vi "GINKGO - MTMP - 20180213A.vi"() -> ()   [LabVIEW 2015]
uses:
  <vilib>/rvi/interface/nirviMethod/nirviMethod.xnode
  <vilib>/rvi/interface/nirviCloseFPGA/nirviCloseFPGA.xnode
  <vilib>/rvi/interface/nirviReadWriteControl/nirviReadWriteControl.xnode
  <vilib>/rvi/interface/nirviOpenFPGA/nirviOpenFPGA.xnode
  <vilib>/rvi/interface/Simulation/niFpgaSimulationCallBeginRW.vi
  <vilib>/rvi/errors/niLvFpgaAdjustHostInterfaceError.vi
  <vilib>/rvi/errors/niLvFpgaMergeErrorWithErrorCode.vi
  <vilib>/FPGAPlugInAG/Dynamic/niLvFpga_Abort_Dynamic.vi
  <vilib>/FPGAPlugInAG/Dynamic/niLvFpga_Reset_Dynamic.vi
  <vilib>/FPGAPlugInAG/Dynamic/niLvFpga_Run_Dynamic.vi
  NiFpgaLv.dll
  <vilib>/Utility/error.llb/Error Cluster From Error Code.vi
  <vilib>/FPGAPlugInAG/Dynamic/niLvFpga_Close_Dynamic.vi
  <vilib>/FPGAPlugInAG/Dynamic/niLvFpga_ReadFifo_Dynamic.vi
  <vilib>/rvi/interface/common/dynamic/niFpgaDynamicAddResources.vi
  <vilib>/FPGAPlugInAG/Dynamic/niLvFpga_StopFifo_Dynamic.vi
  Controls/Save picture camera.vi
  <vilib>/vision/NI_Vision_Development_Module.lvlib
  Global Variable/GV_Z axis.vi
  Global Variable/GV_Lock State.vi
  <vilib>/FPGAPlugInAG/Dynamic/niLvFpga_WriteFifo_Dynamic.vi
  <vilib>/FPGAPlugInAG/Dynamic/niLvFpga_ConfigureFifo_Dynamic.vi
  <vilib>/FPGAPlugInAG/Dynamic/niLvFpga_StartFifo_Dynamic.vi
  FPGA Bitfiles/MiniScan2.2.9_7853R_FPGAControl5_Gcp--B4KBuM.lvbitx
  FPGA/FPGA Control.vi
  FPGA Bitfiles/MiniScan2.2.9_7961R_FPGA796xR2_XT1A-d32QCQ.lvbitx
  FPGA/FPGA 796xR.vi
  FPGA Bitfiles/GINKGO-MTPM_7854R_FPGAControl5_d88-Mrxru6Q.lvbitx
  <vilib>/FPGAPlugInAG/PXI-7854R/niLvFpga_Open_PXI-7854R.vi
  FPGA Bitfiles/GINKGO-MTPM_7975R_FPGA796xR_a2zTekeNlbw.lvbitx
  <vilib>/FPGAPlugInAG/PXIe-7975R/niLvFpga_Open_PXIe-7975R.vi
  <vilib>/FPGAPlugInAG/PXI-7853R/niLvFpga_Open_PXI-7853R.vi
  <vilib>/FPGAPlugInAG/PXIe-7961R/niLvFpga_Open_PXIe-7961R.vi
panel:
  out "波形图表":sgl(graph)=113.25391
  in  "ROI Statistic":bool=TRUE
  out "Mean Value":sgl=113.25391
  out "Variation":sgl=54.35391
  out "Minimal":sgl=32720.0
  out "Maximal":sgl=33176.0
  out "Power Stop":bool=TRUE
  in  "Rolling Queue Flag":bool=TRUE
  out "Total Data Out":u16=13612
  in  "Acq. Start":u16=38 caption="Phase" max=6000 step=1
  in  "Real Back Period":u16=5 min=1
  out "实际深度":u32=8388608
  in  "Map Max.":i32=10000 caption="Max."
  in  "Map Min.":i32=-500 caption="Min."
  out "Scale Value":dbl=0.1 caption="X"
  out "Total Frames":u16=16553
  in  "Max. Min.":cluster{i32, i32}(slide)={429, -176} scale=-500.0..10000.0
  in  "16-bit Display Method":u32(ring)=14 caption="Display Method" items=["Full Dynamic"=12, "Given Range"=14]
  in  "Rolling Average":dbl=2.0 min=1.0 step=1.0
  in  "Rolling":bool=TRUE
  out "User Define Phase":u32=746
  out "Image":T1(plugin-control)
  in  "Controls":T2(tab)
  in  "Start Device":bool
  in  "PMT Shutter Pow.":bool
  out "Overload Dis.":bool=TRUE
  in  "Pulse Number":enum16{"SP", "DP"}(ring)
  in  "Mems Enable":bool
  out "中心偏移":i32
  in  "互相关点数":i32=5
  in  "Calculate Phase shift":bool
  in  "Wave":enum16{"Triangle", "Sine", "Ramp"}(ring)=enum."Sine"
  in  "Interval Dis.":sgl=0.00049965957 min=-10 max=50 format="%.4f"
  in  "stop z stage":bool
  in  "5V":bool
  in  "Voltage Level":dbl=15.0 format="%#.3p"
  in  "Voltage Level 2":dbl=-15.0 caption="Voltage Level" format="%#.3p"
  in  "Source:Output Enabled":bool
  out "Voltage Measurement 2":dbl=-0.0001217159676001422 caption="Voltage Measurement"
  out "Compliance/Limit Reached 2":bool caption="Compliance/Limit Reached"
  out "Voltage Measurement":i8
  out "Compliance/Limit Reached":bool
  in  "MEMS SLOW":dbl(slide)=240000.0 caption="Slow" min=0.0 max=1000000.0 step=100.0 scale=0.0..300000.0 scale format="%#_6p"
  in  "MEMS FAST":dbl(slide) caption="Fast" min=0.0 max=1000000.0 step=100.0 scale=0.0..300000.0 scale format="%#_6p"
  out "Stimulate Time Dis.":u32
  in  "Stimulate Value":dbl=5.0 min=-10.0 max=10.0 format="%#_3f"
  in  "Stimulate Time":u32=500
  out "Stimulate Interval Time":dbl=1.9692307692307693
  in  "Stimulate Interval":u32=10
  in  "Stimulate Enable":bool caption="V.S."
  out "Frame Befor Time":dbl=845778175.0153847
  out "Frame Number":u32=4294967295
  in  "Frames Befor Stimulate":u32
  out "Acq. Sample Rate":dbl=120000000.0 caption="Sanple Rate Divider" format="%#_6p"
  in  "Microscope":enum16{"Miniature", "Benchtop"}(ring)
  in  "Line":u32(ring)=512 caption="Y" items=["8"=8, "16"=16, "32"=32, "64"=64, "128"=128, "256"=256, "512"=512, "1024"=1024, "2048"=2048]
  in  "X Offset":dbl caption="X" format="%#_3f"
  in  "Y Offset":dbl caption="Y" min=-10.0 max=10.0 format="%#_3f"
  in  "X Frequency":dbl(slide)=2600.0 caption="Speed" min=50.0 max=10000.0 step=1.0 scale=0.0..5000.0
  in  "Laser Intensity":dbl(slide)=2.0786516853932584 max=10.0 scale=0.0..5.0
  in  "Phase Shift":u32(slide)=752 caption="Phase" max=15000 step=2 scale=0.0..15000.0
  in  "Point":bool
  in  "PMT1 Sensitivity":dbl(slide)=0.5 min=0.0 max=0.95 step=0.05 scale=0.0..0.95 scale format="%#_3f"
  in  "PMT1 Enable":bool=TRUE
  out "Pixel Dwell":dbl=0.2988 format="%#_3g"
  out "Actual Positon":sgl=11.119017
  out "Actual Laser Intensity":dbl(knob)=0.69488525390625 scale=-10.0..1.0
  in  "PMT2 Switch":bool
  in  "PMT2 Sensitivity":dbl(slide)=0.45 min=0.0 max=0.95 step=0.05 scale=0.0..0.95 scale format="%#_3f"
  in  "File Name":string
  in  "Scale":bool
  in  "XY Home":bool
  in  "XY UP":bool
  in  "XY DOWN":bool
  in  "XY LEFT":bool
  in  "XY RIGHT":bool
  in  "Stop":bool=TRUE
  in  "LIVE":bool
  in  "Save":bool
  in  "Z-Stack":bool
  in  "Pixel/Line":u16(ring)=512 caption="X" items=["8"=8, "16"=16, "32"=32, "64"=64, "128"=128, "256"=256, "512"=512, "1024"=1024, "2048"=2048]
  in  "Gain":enum16{"0dB", "6dB", "12dB"}(ring)
  in  "Coulple":enum16{"AC", "DC"}(ring)=enum."DC"
  in  "Path":path=path "C:/Users/TVS001/Desktop/DATA/20180207/13-zz-gcamp" caption="Images Folder"
  out "Save Frames Dis.":u16=1000
  in  "Save Frames":u16=1000
  in  "ZOOM":u16(ring)=2 items=["User Define", "1X", "1.5X", "2X", "2.5X", "3X", "3.5X", "4X", "4.5X", "5X", "6X"]
  in  "Scan Mode":enum16{"Normal", "Line Scan", "Random Access"}(ring)
  in  "Y Amplitude":dbl=0.6 caption="Y" min=-10.0 max=18.0 format="%0.2p"
  in  "X Amplitude":dbl=0.6 caption="X" min=-10.0 max=18.0 format="%.2p"
  in  "Add Phase":bool
  in  "Move":bool=TRUE
  out "Frame Rate":dbl=5.078125 format="%#_3g"
  out "Ready":u8(slide)=10 scale=0.0..10.0
  in  "Z":bool
  out "Position":sgl=-5.9652176 format="%#_6f"
  in  "Set Zero":bool caption="空白按钮"
  in  "Reset Zero":bool caption="空白按钮"
  in  "Home Z":bool
  in  "Abs. Go":bool
  in  "Abs Pos X":sgl min=-10 max=360 format="%.6f"
  in  "Z Up":bool
  in  "Z Down":bool
  in  "Jog":sgl=0.0005 caption="Z" min=0 max=50 step=0.0001 format="%.4f"
  in  "Frames/Slice":u16=5
  in  "Slices":u16=87
  out "End Dis.":sgl=0.043470383 format="%#_6f"
  out "Start Dis.":sgl format="%#_6f"
  in  "End":bool
  in  "Start":bool
  in  "Restart":bool
  in  "Interval Time":u32=150
  in  "Zoom Standard":dbl[][](array[numeric])=[[10.0, 10.0, 11251.0], [6.66, 6.66, 10603.0], [5.0, 5.0, 10394.0], [4.0, 4.0, 10394.0], [3.34, 3.34, 8602.0], [2.86, 2.86, 10394.0], [2.5, 2.5, 10394.0], [2.222, 2.222, 10394.0], [1.3, 1.3, 8294.0], [0.6, 0.6, 8296.0]]
  in  "Zoom Miniature":dbl[][](array[numeric])=[[14.0, 8.0, 738.0], [12.0, 7.0, 746.0], [9.0, 6.0, 752.0], [7.2, 5.6, 754.0], [5.0, 4.0, 738.0], [5.14, 4.0, 846.0], [4.0, 3.0, 744.0], [3.6, 2.0, 840.0], [3.2, 2.3, 754.0], [3.0, 2.33, 740.0]]
  out "Test Point2":u32
  out "Test Point 3":u32=143394
  out "Test Point":u32
  out "Point/Pixel":i32=36
  in  "Focus Flag":bool
  out "Queue Number":i32=2
  out "Initial Z":bool
  out "Initialization Done":bool=TRUE
  in  "Start Control":bool
  out "Memory":i32(slide) scale=0.0..5000.0
  in  "Resource Name":refnum<k15>="PXI1Slot6"
  in  "Channel Name":string="1" caption="Channel Name 1"
  in  "Current Limit":dbl=0.5 format="%.3p"
  in  "Voltage Level Range":dbl=20.0 format="%.5p"
  in  "Current Limit Range":dbl=1.0 format="%.3p"
  in  "Source Delay (Sec)":dbl=0.1 format="%.3p"
  in  "Channel Name 2":string="2"
  out "Current Measurement 2":dbl=-3.1048749529460624e-06 caption="Current Measurement"
  out "Current Measurement":i16
  out "Actual DDS Ticks":u32=1
  out "Actual DDS Sample Freq":u32=279173
  in  "OUTPUT Value Ticks":u32=44
  in  "DDS Ticks":u32=1
  out "Actual OUTPUT Value Ticks":u32=44
  in  "Random 1D Array":fxp<+/-,32,16>[](array[numeric]) format="%.21g"
  in  "MG17Motor Z":refnum<k7>(container)
  out "Acq. Point Dis.":u16=32
  in  "Divide":enum16{"120M", "60M", "30M", "15M", "7.5M"}(ring)
  out "Nonlinear Acq.":bool=TRUE
  in  "Adapter Module User Data 1":u8
  in  "Adapter Module User Data 0":u8
  in  "Adapter Module User Command":u8=3
  in  "Apply":bool
  in  "HWSerialNum":i32=49871607
  in  "Set Large Scale":dbl=0.5 caption="X"
  in  "Set Small Scale":dbl=0.1 caption="X"
  in  "Set Zero Value":sgl format="%#_6f"
  in  "Fill Fraction":dbl=0.8 min=0.1 max=6.0 step=0.01
  in  "Back Period":u16=5 min=1
  in  "Initial Benchtop Speed":dbl=500.0 caption="Speed" min=50.0 max=10000.0 step=1.0
  in  "Initial Miniature Speed":dbl=2600.0 caption="Speed" min=50.0 max=10000.0 step=1.0
  out "Acq.Point Array":u16[](graph)=[38, 38, 38, 37, 37, 37, 37, 36, 36, 36, 36, 36, 35, 35, 35, 35, 35, 34, 34, 34, 34, 34, 34, 33, 33, 33, 33, 33, 33, 32, 32, 32, 32, 32, 32, 32, 32, 31, 31, 31, 31, 31, 31, 31, 31, 30, 30, 30, 30, 30, 30, 30, 30, 30, 30, 29, 29, 29, 29, 29, 29, 29, 29, 29, 29, 29, 28, 28, 28, 28, 28, 28, 28, 28, 28, 28, 28, 28, 28, 28, 27, 27, 27, 27, 27, 27, 27, 27, 27, 27, 27, 27, 27, 27, 27, 27, 26, 26, 26, 26, 26, 26, 26, 26, 26, 26, 26, 26, 26, 26, 26, 26, 26, 26, 26, 26, 26, 25, 25, 25, 25, 25, 25, 25, 25, 25, 25, 25, 25, 25, 25, 25, 25, 25, 25, 25, 25, 25, 25, 25, 25, 25, 25, 25, 24, 24, 24, 24, 24, 24, 24, 24, 24, 24, 24, 24, 24, 24, 24, 24, 24, 24, 24, 24, 24, 24, 24, 24, 24, 24, 24, 24, 24, 24, 24, 24, 24, 24, 24, 24, 24, 24, 24, 24, 24, 24, 24, 23, 23, 23, 23, 23, 23, 23, 23, 23, 23, 23, 23, 23, 23, 23, 23, 23, 23, 23, 23, 23, 23, 23, 23, 23, 23, 23, 23, 23, 23, 23, 23, 23, 23, 23, 23, 23, 23, 23, 23, 23, 23, 23, 23, 23, 23, 23, 23, 23, 23, 23, 23, 23, 23, 23, 23, 23, 23, 23, 23, 23, 23, 23, 23, 23, 23, 23, 23, 23, 23, 23, 23, 23, 23, 23, 23, 23, 23, 23, 23, 23, 23, 23, 23, 23, 23, 23, 23, 23, 23, 23, 23, 23, 23, 23, 23, 23, 23, 23, 23, 23, 23, 23, 23, 23, 23, 23, 23, 23, 23, 23, 23, 23, 23, 23, 23, 23, 23, 23, 23, 23, 23, 23, 23, 23, 23, 23, 23, 23, 23, 23, 23, 23, 23, 23, 23, 23, 23, 24, 24, 24, 24, 24, 24, 24, 24, 24, 24, 24, 24, 24, 24, 24, 24, 24, 24, 24, 24, 24, 24, 24, 24, 24, 24, 24, 24, 24, 24, 24, 24, 24, 24, 24, 24, 24, 24, 24, 24, 24, 24, 24, 25, 25, 25, 25, 25, 25, 25, 25, 25, 25, 25, 25, 25, 25, 25, 25, 25, 25, 25, 25, 25, 25, 25, 25, 25, 25, 25, 26, 26, 26, 26, 26, 26, 26, 26, 26, 26, 26, 26, 26, 26, 26, 26, 26, 26, 26, 26, 26, 27, 27, 27, 27, 27, 27, 27, 27, 27, 27, 27, 27, 27, 27, 27, 27, 28, 28, 28, 28, 28, 28, 28, 28, 28, 28, 28, 28, 28, 28, 29, 29, 29, 29, 29, 29, 29, 29, 29, 29, 29, 30, 30, 30, 30, 30, 30, 30, 30, 30, 30, 31, 31, 31, 31, 31, 31, 31, 31, 32, 32, 32, 32, 32, 32, 32, 32, 33, 33, 33, 33, 33, 33, 34, 34, 34, 34, 34, 34, 35, 35, 35, 35, 35, 36, 36, 36, 36, 36, 37, 37, 37, 37, 38, 38, 38]
  out "Init Data Out":u16[](array[numeric])=[38, 38, 38, 37, 37, 37, 37, 36, 36, 36, 36, 36, 35, 35, 35, 35, 35, 34, 34, 34, 34, 34, 34, 33, 33, 33, 33, 33, 33, 32, 32, 32, 32, 32, 32, 32, 32, 31, 31, 31, 31, 31, 31, 31, 31, 30, 30, 30, 30, 30, 30, 30, 30, 30, 30, 29, 29, 29, 29, 29, 29, 29, 29, 29, 29, 29, 28, 28, 28, 28, 28, 28, 28, 28, 28, 28, 28, 28, 28, 28, 27, 27, 27, 27, 27, 27, 27, 27, 27, 27, 27, 27, 27, 27, 27, 27, 26, 26, 26, 26, 26, 26, 26, 26, 26, 26, 26, 26, 26, 26, 26, 26, 26, 26, 26, 26, 26, 25, 25, 25, 25, 25, 25, 25, 25, 25, 25, 25, 25, 25, 25, 25, 25, 25, 25, 25, 25, 25, 25, 25, 25, 25, 25, 25, 24, 24, 24, 24, 24, 24, 24, 24, 24, 24, 24, 24, 24, 24, 24, 24, 24, 24, 24, 24, 24, 24, 24, 24, 24, 24, 24, 24, 24, 24, 24, 24, 24, 24, 24, 24, 24, 24, 24, 24, 24, 24, 24, 23, 23, 23, 23, 23, 23, 23, 23, 23, 23, 23, 23, 23, 23, 23, 23, 23, 23, 23, 23, 23, 23, 23, 23, 23, 23, 23, 23, 23, 23, 23, 23, 23, 23, 23, 23, 23, 23, 23, 23, 23, 23, 23, 23, 23, 23, 23, 23, 23, 23, 23, 23, 23, 23, 23, 23, 23, 23, 23, 23, 23, 23, 23, 23, 23, 23, 23, 23, 23, 23, 23, 23, 23, 23, 23, 23, 23, 23, 23, 23, 23, 23, 23, 23, 23, 23, 23, 23, 23, 23, 23, 23, 23, 23, 23, 23, 23, 23, 23, 23, 23, 23, 23, 23, 23, 23, 23, 23, 23, 23, 23, 23, 23, 23, 23, 23, 23, 23, 23, 23, 23, 23, 23, 23, 23, 23, 23, 23, 23, 23, 23, 23, 23, 23, 23, 23, 23, 23, 24, 24, 24, 24, 24, 24, 24, 24, 24, 24, 24, 24, 24, 24, 24, 24, 24, 24, 24, 24, 24, 24, 24, 24, 24, 24, 24, 24, 24, 24, 24, 24, 24, 24, 24, 24, 24, 24, 24, 24, 24, 24, 24, 25, 25, 25, 25, 25, 25, 25, 25, 25, 25, 25, 25, 25, 25, 25, 25, 25, 25, 25, 25, 25, 25, 25, 25, 25, 25, 25, 26, 26, 26, 26, 26, 26, 26, 26, 26, 26, 26, 26, 26, 26, 26, 26, 26, 26, 26, 26, 26, 27, 27, 27, 27, 27, 27, 27, 27, 27, 27, 27, 27, 27, 27, 27, 27, 28, 28, 28, 28, 28, 28, 28, 28, 28, 28, 28, 28, 28, 28, 29, 29, 29, 29, 29, 29, 29, 29, 29, 29, 29, 30, 30, 30, 30, 30, 30, 30, 30, 30, 30, 31, 31, 31, 31, 31, 31, 31, 31, 32, 32, 32, 32, 32, 32, 32, 32, 33, 33, 33, 33, 33, 33, 34, 34, 34, 34, 34, 34, 35, 35, 35, 35, 35, 36, 36, 36, 36, 36, 37, 37, 37, 37, 38, 38, 38]
  out "x amp. new":dbl
  out "y amp. new":dbl
  in  "Add Random Access":bool
  out "x offset new":i16=-7638
  out "y offset new":i16=-4030
  in  "All Random Array":fxp<+/-,32,16>[][](array[numeric])
  in  "Clear Array":bool
  out "Random Phase":u32=12 caption="Phase" max=6000 step=1
  # "File Name"
  # "File Path"
  # "Save Frames"
  # "Microscope"
  # "Scan Mode"
  # "PMT1"
  # "PMT2"
  # "Frame Size"
  # "Gain"
  # "Scan Speed"
  # "Hz"
  # "V"
  # "V"
  # "Rate"
  # "Frame Rate"
  # "μs"
  # "Hz"
  # "Pixel Dwell"
  # "XY"
  # "Z"
  # "Zoom"
  # "Point"
  # "Amplitude"
  # "V"
  # "V"
  # "Phase"
  # "Laser"
  # "Intensity Map"
  # "Recent Z"
  # "Frames Before"
  # "s"
  # "Stimulate Interval"
  # "s"
  # "ms"
  # "Stimulate Time"
  # "V"
  # "Stimulate Intensity"
  # "Mode Switch"
  # "MEMS Filter"
  # "Acquisition Mode"
  # "Image Settings"
  # "Magnification"
  # "Save Settings"
  # "Position Settings"
  # "Detection Settings"
  # "Z-scan Settings"
  # "Vision Stimulate Settings"
  # "X"
  # "Y"
  # "Phase"
  # "1X"
  # "1.5X"
  # "2X"
  # "2.5X"
  # "3X"
  # "3.5X"
  # "4X"
  # "4.5X"
  # "5X"
  # "6X"
  # "X"
  # "Y"
  # "Phase"
  # "1X"
  # "1.5X"
  # "2X"
  # "2.5X"
  # "3X"
  # "3.5X"
  # "4X"
  # "4.5X"
  # "5X"
  # "6X"
  # "40859011"
  # "83856379"
  # "AO0 -- X-Miniature  \nAO1 -- Y-Miniature\nAO2 -- Laser Intensity\nAO3 -- PMT1\nAO4 -- PMT2 \nAO5 -- \nAO6 -- X-Benchtop\nAO7 -- Y-Benchtop\n\nAI0  -- Actual Laser Intensity"
  # "DIO0 -- Acqusition  \nDIO1 -- VSYNC\nDIO2 -- HSYNC \nDIO3 -- Laser Shutter\nDIO4 -- MEMS FAST Filter\nDIO5 -- MEMS SLOW Filter\nDIO6 -- PMT Shutter\nDIO7 -- PMT Shutter Pow.\nDIO8 -- Shock Detection \nDIO9 -- Foot-plate LIVE Detection"
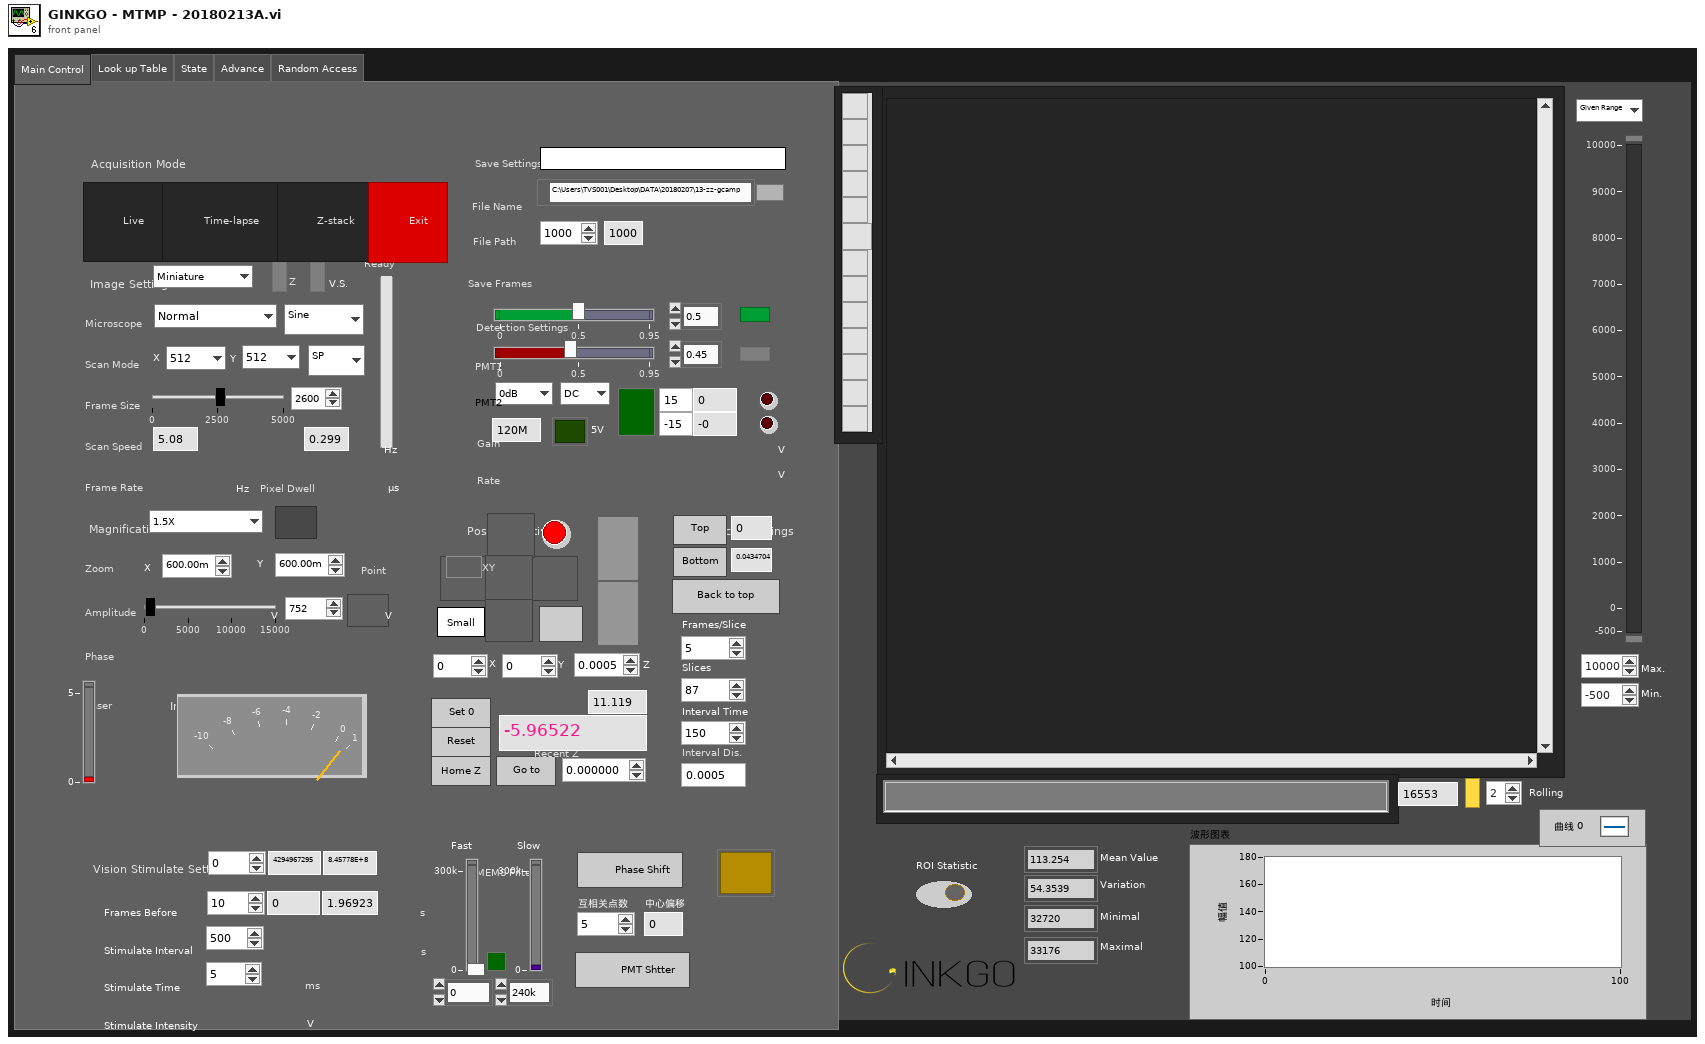
[diagram p1: front panel]
types:
  T1 = typedef "IMAQ Image.ctl" = refnum<image>
  T2 = enum32{"Main Control", "Look up Table", "State", "Advance", "Random Access"}
  T3 = typedef "Image Type" = u32
  T4 = enum8{"Enabled", "Disabled", "Disabled and Grayed Out"}
  T5 = cluster{"Global Rectangle":i32[], "Contours":cluster{"Contour Type":u32, "ROI Type":u32, "Points":i32[]}[]}
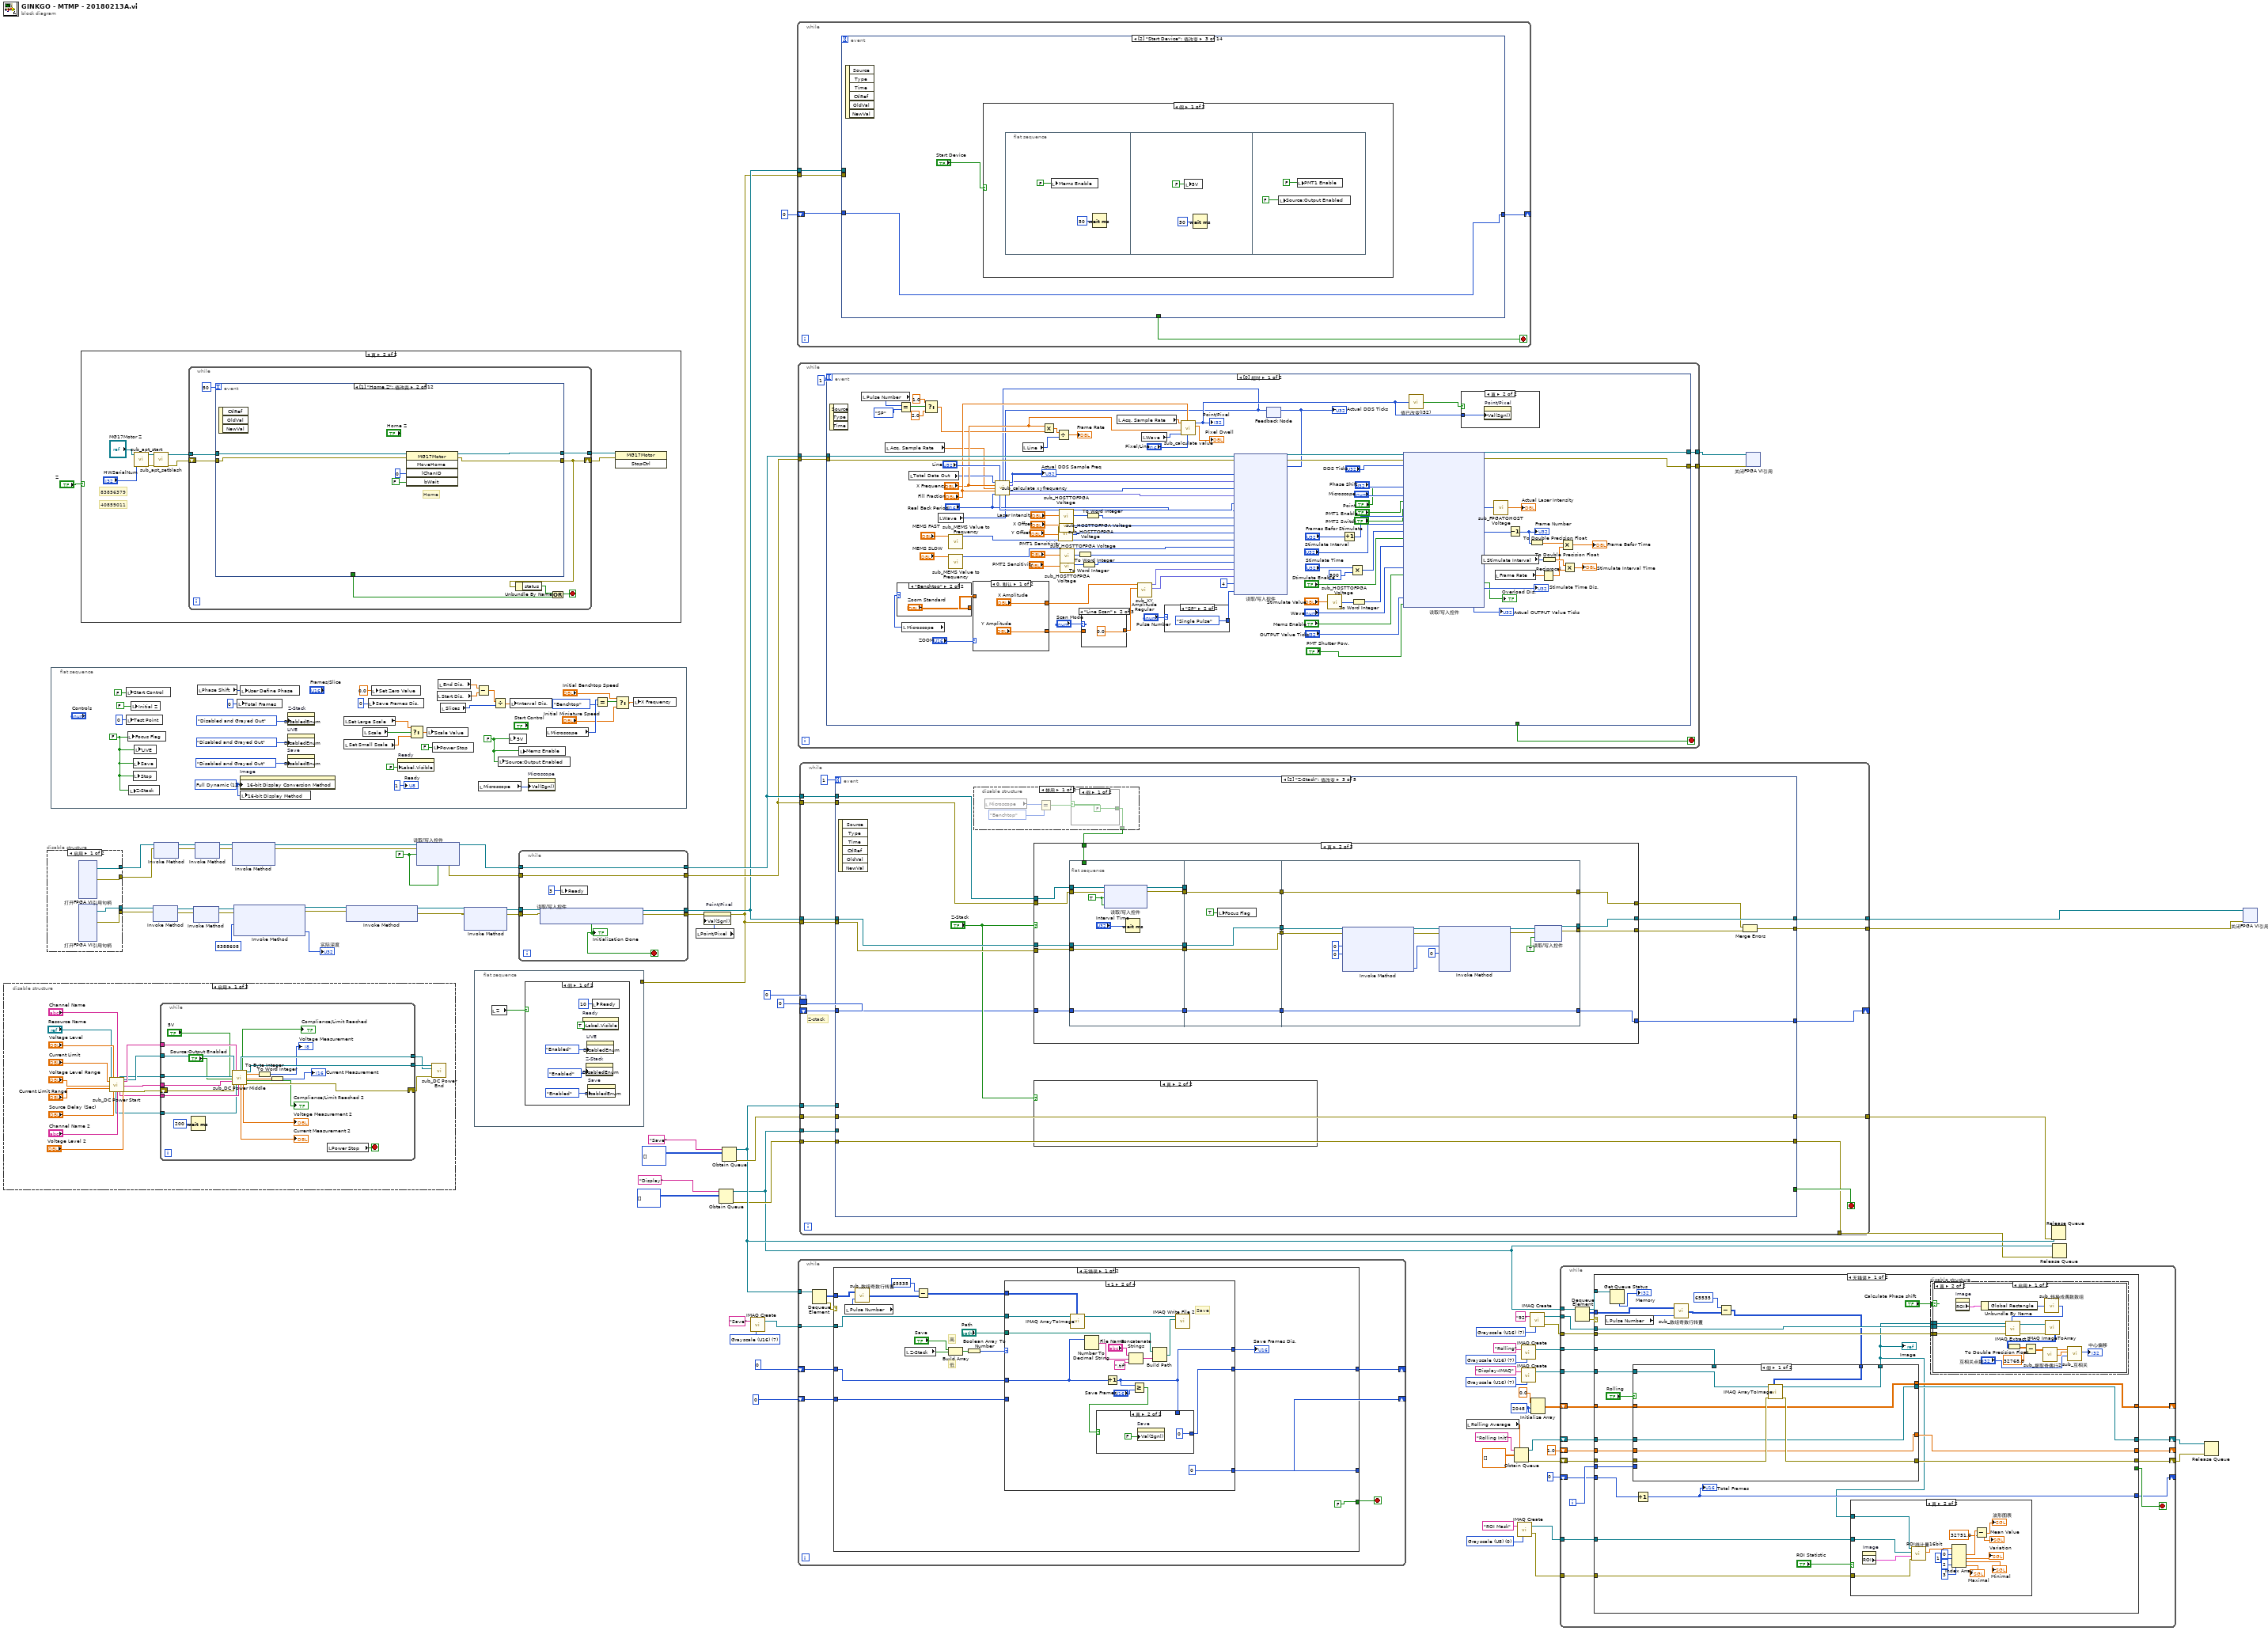
[diagram p0: block diagram]
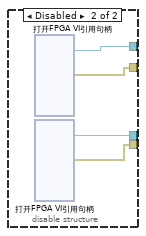
[diagram p2: hidden frame]
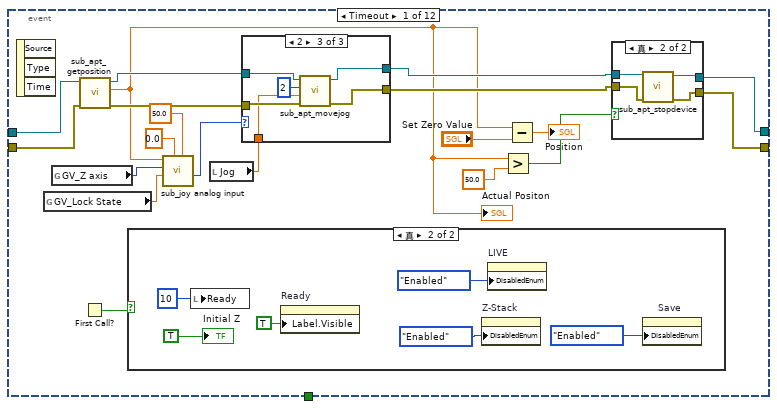
[diagram p4: hidden frame]
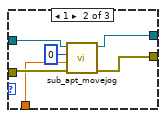
[diagram p6: hidden frame]
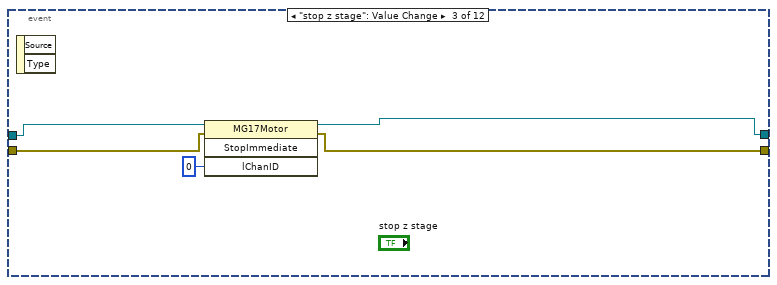
[diagram p9: hidden frame]
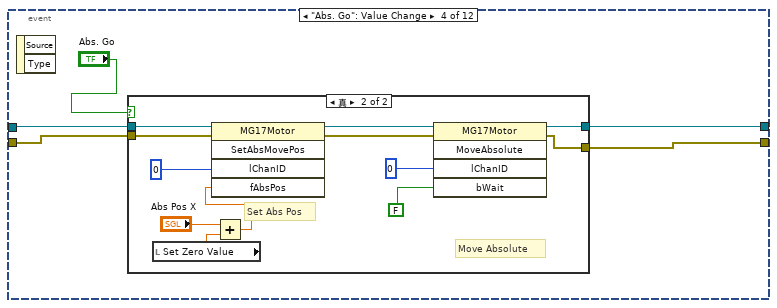
[diagram p10: hidden frame]
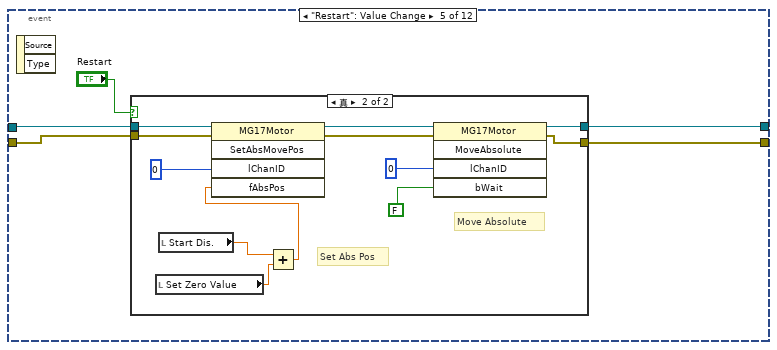
[diagram p12: hidden frame]
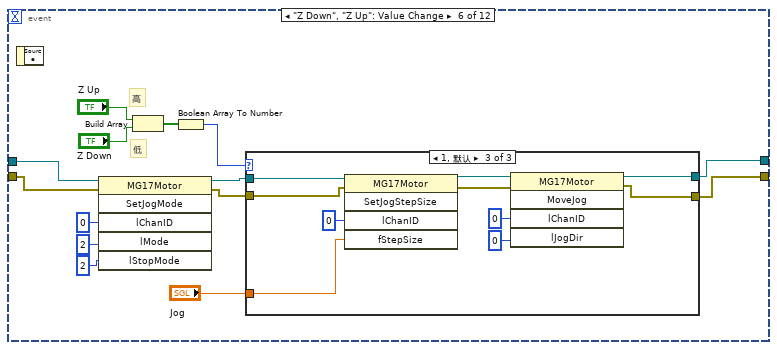
[diagram p14: hidden frame]
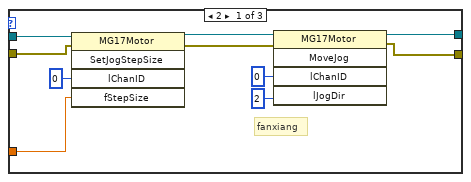
[diagram p15: hidden frame]
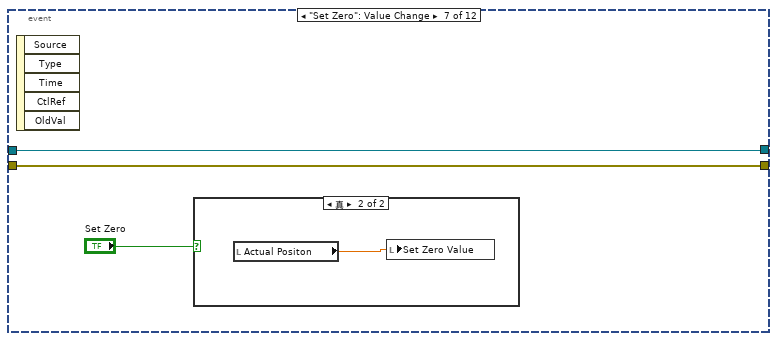
[diagram p17: hidden frame]
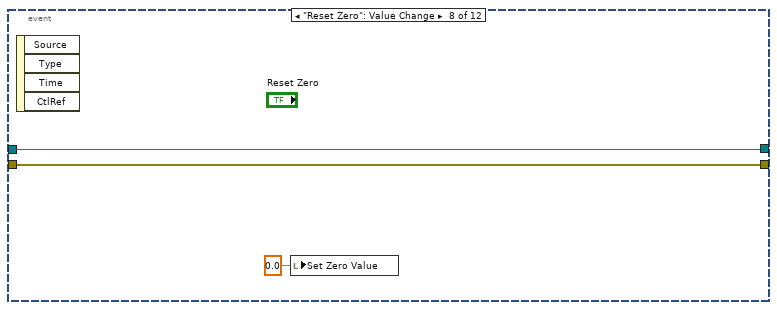
[diagram p19: hidden frame]
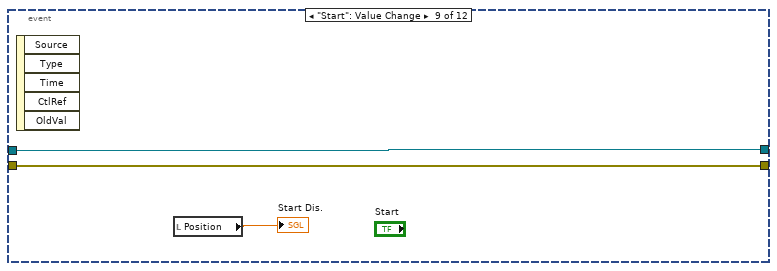
[diagram p20: hidden frame]
diagram:
  w3 = T3 0 items=["Grayscale (U8)", "Grayscale (I16)", "Grayscale (SGL)", "Complex (CSG)", "RGB (U32)", "HSL (U32)", "RGB (U64)", "Grayscale (U16)"] ("Image Type")
  w9 = T3 7 items=["Grayscale (U8)", "Grayscale (I16)", "Grayscale (SGL)", "Complex (CSG)", "RGB (U32)", "HSL (U32)", "RGB (U64)", "Grayscale (U16)"] ("Image Type")
  w15 = T3 7 items=["Grayscale (U8)", "Grayscale (I16)", "Grayscale (SGL)", "Complex (CSG)", "RGB (U32)", "HSL (U32)", "RGB (U64)", "Grayscale (U16)"] ("Image Type")
  w28 = T3 7 items=["Grayscale (U8)", "Grayscale (I16)", "Grayscale (SGL)", "Complex (CSG)", "RGB (U32)", "HSL (U32)", "RGB (U64)", "Grayscale (U16)"] ("Image Type")
  w38 = 2048 ("维数大小")
  w35 = T3 7 items=["Grayscale (U8)", "Grayscale (I16)", "Grayscale (SGL)", "Complex (CSG)", "RGB (U32)", "HSL (U32)", "RGB (U64)", "Grayscale (U16)"] ("Image Type")
  w49 = FALSE ("Enable")
  n1 = disable-structure shown="启用" {
    frame Enabled {
      n2 = call "sub_DC Power Start.vi"("IVI引用句柄输入"="Resource Name", "Current Limit"="Current Limit", "Voltage Level Range"="Voltage Level Range", "Current Limit Range"="Current Limit Range", "Voltage Level"="Voltage Level", "Source Delay (Sec)"="Source Delay (Sec)", "Channel Name"="Channel Name", "Channel Name 2"="Channel Name 2", "Voltage Level 2"="Voltage Level 2") -> ("instrument handle out 2"=w81:refnum<k15>, "instrument handle out"=w88:refnum<k15>, "Channel Name 6"=w82:string, "IVI引用句柄输出"=w96:refnum<k15>, "Channel Name 4"=w97:string, "Channel Name 3"=w90:string, "错误输出"=w87:errorcluster)  [unwired: 4 in]
      n3 = while {
        tunnel: w97 -> [w121]
        tunnel: w90 -> [w120]
        tunnel: [w119] -> w89
        shift-right: [w118] -> w86
        shift-left: w87 -> [w115]
        tunnel: w88 -> [w114]
        tunnel: w96 -> [w116]
        tunnel: [w117] -> w98
        tunnel: w82 -> [w104]
        tunnel: w81 -> [w103]
        stop <- w105 stop-if-true
        n4 = Wait (ms)(milliseconds to wait=u32 200 ("等待时间（毫秒）")) -> ()  [unwired: 1 out]
        n5 = call "sub_DC Power Middle.vi"("IVI引用句柄输入"=w116, "instrument handle out"=w114, "5V"="5V", "Source:Output Enabled"="Source:Output Enabled", "Channel Name 3"=w120, "错误输入（无错误）"=w115, "Channel Name 4"=w121, "instrument handle out 2"=w103, "Channel Name 5"=w104) -> ("instrument handle out 3"=w119:refnum<k15>, "Current Measurement 2"=→"Current Measurement 2":dbl, "Compliance/Limit Reached"=→"Compliance/Limit Reached":bool, "Voltage Measurement 2"=→"Voltage Measurement 2":dbl, "IVI引用句柄输出"=w117:refnum<k15>, "Voltage Measurement"=w111:dbl, "Current Measurement"=w110:dbl, "Compliance/Limit Reached 2"=→"Compliance/Limit Reached 2":bool, "错误输出"=w118:errorcluster)  [unwired: 2 in]
        n6 = To Byte Integer(number=w111) -> (8bit integer=→"Voltage Measurement":i8)
        n7 = To Word Integer(number=w110) -> (16bit integer=→"Current Measurement":i16)
        n8 = local read "Power Stop"() -> (w105:bool)
      }
      n9 = call "sub_DC Power End.vi"("错误输入（无错误）"=w86, "instrument handle out"=w89, "IVI引用句柄输入"=w98) -> ()  [unwired: 9 in]
    }
    frame Disabled {
    }
  }
  n10 = disable-structure shown="启用" {
    disable-tunnel: [w125 w129] -> w80
    disable-tunnel: [w124 w128] -> w79
    disable-tunnel: [w123 w126] -> w78
    disable-tunnel: [w122 w127] -> w77
    frame Enabled {
      n11 = xnode "打开FPGA VI引用句柄"() -> ("FPGA VI引用输出"=w125:refnum<k20>, "错误输出"=w124:errorcluster)  [unwired: 2 in]
      n12 = xnode "打开FPGA VI引用句柄"() -> ("FPGA VI引用输出"=w122:refnum<k20>, "错误输出"=w123:errorcluster)  [unwired: 2 in]
    }
    frame Disabled {
      n13 = xnode "打开FPGA VI引用句柄"() -> ("FPGA VI引用输出"=w129:refnum<k20>, "错误输出"=w128:errorcluster)  [unwired: 2 in]
      n14 = xnode "打开FPGA VI引用句柄"() -> ("FPGA VI引用输出"=w127:refnum<k20>, "错误输出"=w126:errorcluster)  [unwired: 2 in]
    }
  }
  n15 = flat-sequence {
    frame #0 {
      w143 = FALSE ("Focus")
      w151 = u32 12 items=["Default"=10, "Most Significant Bits"=11, "Full Dynamic"=12, "Downshift"=13, "Given Range"=14, "90% Dynamic"=15, "Given Percent Range"=16] ("16-bit Display Mapping:Conversion Method")
      w158 = FALSE ("Focus")
      n16 = local write "Start Control"(FALSE ("Initial")) -> ()
      n17 = local write "Test Point"(u32 0 ("Test Point")) -> ()
      n18 = local write "Focus Flag"(w158) -> ()
      n19 = local write "Z-Stack"(w158) -> ()
      n20 = local write "Initial Z"(FALSE ("Initial")) -> ()
      n21 = local write "Save"(w158) -> ()
      n22 = local write "Stop"(w158) -> ()
      n23 = local write "LIVE"(w158) -> ()
      n24 = local read "Phase Shift"() -> (w144:u32)
      n25 = local write "Total Frames"(u16 0 ("Total Frames")) -> ()
      n26 = property on="Image" class="ImageControl"("16-bit Display Conversion Method"=w151) -> ()  [unwired: 2 in, 2 out]
      n27 = local write "User Define Phase"(w144) -> ()
      n28 = local write "16-bit Display Method"(w151) -> ()
      n29 = property on="LIVE" class="Bool (严格)"("DisabledEnum"=T4."Disabled and Grayed Out" ("禁用")) -> ()  [unwired: 2 in, 2 out]
      n30 = property on="Save" class="Bool (严格)"("DisabledEnum"=T4."Disabled and Grayed Out" ("禁用")) -> ()  [unwired: 2 in, 2 out]
      n31 = property on="Z-Stack" class="Bool (严格)"("DisabledEnum"=T4."Disabled and Grayed Out" ("禁用")) -> ()  [unwired: 2 in, 2 out]
      n32 = local read "Set Large Scale"() -> (w150:dbl)
      n33 = local read "Set Small Scale"() -> (w149:dbl)
      n34 = local read "Scale"() -> (w148:bool)
      n35 = local write "Save Frames Dis."(u16 0 ("Save Frames Dis.")) -> ()
      n36 = local write "Set Zero Value"(sgl 0.0 ("Set Zero Value")) -> ()
      n37 = property on="Ready" class="Slide (严格)"("Label.Visible"=FALSE ("标签.可见")) -> ()  [unwired: 2 in, 2 out]
      n38 = Select(t=w150, s=w148, f=w149) -> (s? t:f=w147:dbl)
      n39 = local write "Scale Value"(w147) -> ()
      n40 = local write "Power Stop"(FALSE ("Power Stop")) -> ()
      n41 = local read "Start Dis."() -> (w140:sgl)
      n42 = local read "End Dis."() -> (w139:sgl)
      n43 = local read "Slices"() -> (w138:u16)
      n44 = Subtract(x=w139, y=w140) -> (x-y=w141:sgl)
      n45 = local read "Microscope"() -> (w137:enum16{"Miniature", "Benchtop"})
      n46 = Divide(x=w141, y=w138) -> (x/y=w142:sgl)
      n47 = local write "Source:Output Enabled"(w143) -> ()
      n48 = local write "5V"(w143) -> ()
      n49 = local write "Interval Dis."(w142) -> ()
      n50 = local write "Mems Enable"(w143) -> ()
      n51 = property on="Microscope" class="Enum (严格)"("Val(Sgnl)"=w137) -> ()  [unwired: 2 in, 2 out]
      n52 = local read "Microscope"() -> (w135:enum16{"Miniature", "Benchtop"})
      n53 = Equal?(x=w135, y=enum16{"Miniature", "Benchtop"}."Benchtop") -> (x = y?=w134:bool)
      n54 = Select(t="Initial Benchtop Speed", s=w134, f="Initial Miniature Speed") -> (s? t:f=w132:dbl)
      n55 = local write "X Frequency"(w132) -> ()
      "Ready" <- u8 1 ("Process")
    }
  }
  n56 = case shown="真" "Z" {
    frame False {
    }
    frame True {
      # "40859011"
      # "83856379"
      n57 = call "sub_apt_start.vi"("HWSerialNum"="HWSerialNum", "引用"="MG17Motor Z") -> ("错误输出"=w166:errorcluster, "引用输出"=w167:refnum<k7>)  [unwired: 8 in]
      n58 = call "sub_apt_setblash.vi"("错误输入（无错误）"=w166, "引用"=w167) -> ("错误输出"=w164:errorcluster, "引用输出"=w165:refnum<k7>)  [unwired: 8 in]
      n59 = while {
        shift-right: [w173] -> w168
        shift-left: w164 -> [w176]
        tunnel: w165 -> [w177]
        tunnel: [w175] -> w169
        stop <- w171 stop-if-true
        n60 = event shown="[1] \"Home Z\": 值改变" {
          selector: _ -> [_ _ _ _ _ _ _ _ _ _ _ _]
          dyn-events: _ -> [_ _ _ _ _ _ _ _ _ _ _ _]
          timeout: 50 -> [_ _ _ _ _ _ _ _ _ _ _ _]
          tunnel: w177 -> [w190 w225 w233 w239 w258 w278 w311 w315 w318 w321 w324 w357]
          tunnel: w176 -> [w189 w224 w232 w238 w257 w277 w310 w314 w317 w320 w323 w356]
          tunnel: [w195 w227 w231 w237 w256 w286 w311 w315 w318 w321 w333 w357] -> w175
          tunnel: [w194 w226 w230 w236 w255 w285 w310 w314 w317 w320 w332 w356] -> w173
          tunnel: [_ _ _ _ _ _ _ _ _ _ _ TRUE ("Stop")] -> w170
          event Timeout {
            n61 = event-data() -> ()  [unwired: 1 in, 3 out]
            n62 = global read "GV_Lock State.vi" "GV_Lock State"() -> (w179:dbl)
            n63 = global read "GV_Z axis.vi" "GV_Z axis"() -> (w180:i32)
            n64 = call "sub_apt_getposition.vi"("错误输入（无错误）"=w189, "引用"=w190) -> ("错误输出"=w186:errorcluster, "GetPosition_Position"=w181:sgl, "引用输出"=w187:refnum<k7>)  [unwired: 7 in]
            "Actual Positon" <- w181
            n65 = First Call?() -> (First Call?: T/F=w193:bool)
            n66 = case shown="真" w193 {
              frame False {
              }
              frame True {
                n67 = local write "Ready"(u8 10 ("Process")) -> ()
                n68 = property on="Ready" class="Slide (严格)"("Label.Visible"=TRUE ("标签.可见")) -> ()  [unwired: 2 in, 2 out]
                n69 = property on="Z-Stack" class="Bool (严格)"("DisabledEnum"=T4."Enabled" ("禁用")) -> ()  [unwired: 2 in, 2 out]
                n70 = property on="LIVE" class="Bool (严格)"("DisabledEnum"=T4."Enabled" ("禁用")) -> ()  [unwired: 2 in, 2 out]
                n71 = property on="Save" class="Bool (严格)"("DisabledEnum"=T4."Enabled" ("禁用")) -> ()  [unwired: 2 in, 2 out]
                "Initial Z" <- TRUE ("Initial")
              }
            }
            n72 = call "sub_joy analog input.vi"("上限"=50.0 ("Displacement"), "下限"=0.0 ("Displacement"), "lock输入奇偶"=w179, "x"=w180, "Displacement"=w181) -> ("x state"=w182:i32)  [unwired: 5 in, 1 out]
            n73 = local read "Jog"() -> (w178:sgl)
            n74 = case shown="2" w182 {
              tunnel: [w199 w202 w208] -> w188
              tunnel: w187 -> [w199 w205 w211]
              tunnel: w186 -> [w198 w204 w210]
              tunnel: [w198 w203 w209] -> w185
              tunnel: w178 -> [_ w201 w207]
              frame 0, Default {
              }
              frame 1 {
                n75 = call "sub_apt_movejog.vi"("错误输入（无错误）"=w204, "Rel. Pos Y"=w201, "lJogDir"=0, "引用"=w205) -> ("error out"=w203:errorcluster, "MG17Motor Y"=w202:refnum<k7>)  [unwired: 6 in]
              }
              frame 2 {
                n76 = call "sub_apt_movejog.vi"("错误输入（无错误）"=w210, "Rel. Pos Y"=w207, "lJogDir"=2, "引用"=w211) -> ("error out"=w209:errorcluster, "MG17Motor Y"=w208:refnum<k7>)  [unwired: 6 in]
              }
            }
            n77 = Greater?(x=w181, y=sgl 50.0) -> (0:w196:bool)
            n78 = Subtract(x=w181, y="Set Zero Value") -> (x-y=→"Position":sgl)
            n79 = case shown="真" w196 {
              tunnel: w188 -> [w219 w223]
              tunnel: w185 -> [w218 w222]
              tunnel: [w219 w221] -> w195
              tunnel: [w218 w220] -> w194
              frame False {
              }
              frame True {
                n80 = call "sub_apt_stopdevice.vi"("错误输入（无错误）"=w222, "引用"=w223) -> ("错误输出"=w220:errorcluster, "引用输出"=w221:refnum<k7>)  [unwired: 8 in]
              }
            }
          }
          event "Home Z": Value Change {
            # "Home"
            n81 = event-data() -> ()  [unwired: 1 in, 3 out]
            n82 = invoke class="MG17Motor" method="MoveHome"(reference=w225, error in=w224, "lChanID"=0, "bWait"=FALSE) -> (reference out=w227:refnum<k7>, error out=w226:errorcluster)  [unwired: 1 in, 3 out]
          }
          event "stop z stage": Value Change {
            n83 = event-data() -> ()  [unwired: 1 in, 2 out]
            n84 = invoke class="MG17Motor" method="StopImmediate"(reference=w233, error in=w232, "lChanID"=0) -> (reference out=w231:refnum<k7>, error out=w230:errorcluster)  [unwired: 1 in, 2 out]
          }
          event "Abs. Go": Value Change {
            n85 = event-data() -> ()  [unwired: 1 in, 2 out]
            n86 = case shown="真" "Abs. Go" {
              tunnel: w239 -> [w241 w250]
              tunnel: w238 -> [w240 w249]
              tunnel: [w241 w246] -> w237
              tunnel: [w240 w245] -> w236
              frame False {
              }
              frame True {
                # "Set Abs Pos"
                # "Move Absolute"
                n87 = local read "Set Zero Value"() -> (w243:sgl)
                n88 = Add(x="Abs Pos X", y=w243) -> (x+y=w242:sgl)
                n89 = invoke class="MG17Motor" method="SetAbsMovePos"(reference=w250, error in=w249, "lChanID"=0, "fAbsPos"=w242) -> (reference out=w248:refnum<k7>, error out=w247:errorcluster)  [unwired: 1 in, 3 out]
                n90 = invoke class="MG17Motor" method="MoveAbsolute"(reference=w248, error in=w247, "lChanID"=0, "bWait"=FALSE) -> (reference out=w246:refnum<k7>, error out=w245:errorcluster)  [unwired: 1 in, 3 out]
              }
            }
          }
          event "Restart": Value Change {
            n91 = event-data() -> ()  [unwired: 1 in, 2 out]
            n92 = case shown="真" "Restart" {
              tunnel: w258 -> [w260 w269]
              tunnel: w257 -> [w259 w268]
              tunnel: [w260 w265] -> w256
              tunnel: [w259 w264] -> w255
              frame False {
              }
              frame True {
                # "Set Abs Pos"
                # "Move Absolute"
                n93 = local read "Set Zero Value"() -> (w263:sgl)
                n94 = local read "Start Dis."() -> (w262:sgl)
                n95 = Add(x=w262, y=w263) -> (x+y=w261:sgl)
                n96 = invoke class="MG17Motor" method="SetAbsMovePos"(reference=w269, error in=w268, "lChanID"=0, "fAbsPos"=w261) -> (reference out=w267:refnum<k7>, error out=w266:errorcluster)  [unwired: 1 in, 3 out]
                n97 = invoke class="MG17Motor" method="MoveAbsolute"(reference=w267, error in=w266, "lChanID"=0, "bWait"=FALSE) -> (reference out=w265:refnum<k7>, error out=w264:errorcluster)  [unwired: 1 in, 3 out]
              }
            }
          }
          event "Z Down", "Z Up": Value Change {
            # "低"
            # "高"
            n98 = event-data() -> ()  [unwired: 1 in, 1 out]
            n99 = invoke class="MG17Motor" method="SetJogMode"(reference=w278, error in=w277, "lChanID"=0, "lMode"=2, "lStopMode"=2) -> (reference out=w280:refnum<k7>, error out=w279:errorcluster)  [unwired: 1 in, 4 out]
            n100 = Build Array("Z Up", "Z Down") -> (w282:bool[])
            n101 = Boolean Array To Number(Boolean array=w282) -> (number=w281:u32)
            n102 = case shown="1, 默认" w281 {
              tunnel: w280 -> [w296 w298 w308]
              tunnel: [w294 w298 w306] -> w286
              tunnel: w279 -> [w291 w297 w303]
              tunnel: [w289 w297 w301] -> w285
              tunnel: "Jog" -> [w287 _ w299]
              frame 2 {
                # "fanxiang"
                n103 = invoke class="MG17Motor" method="SetJogStepSize"(reference=w296, error in=w291, "lChanID"=0, "fStepSize"=w287) -> (reference out=w295:refnum<k7>, error out=w290:errorcluster)  [unwired: 1 in, 3 out]
                n104 = invoke class="MG17Motor" method="MoveJog"(reference=w295, error in=w290, "lChanID"=0, "lJogDir"=2) -> (reference out=w294:refnum<k7>, error out=w289:errorcluster)  [unwired: 1 in, 3 out]
              }
              frame 0 {
              }
              frame 1, Default {
                n105 = invoke class="MG17Motor" method="SetJogStepSize"(reference=w308, error in=w303, "lChanID"=0, "fStepSize"=w299) -> (reference out=w307:refnum<k7>, error out=w302:errorcluster)  [unwired: 1 in, 3 out]
                n106 = invoke class="MG17Motor" method="MoveJog"(reference=w307, error in=w302, "lChanID"=0, "lJogDir"=0) -> (reference out=w306:refnum<k7>, error out=w301:errorcluster)  [unwired: 1 in, 3 out]
              }
            }
          }
          event "Set Zero": Value Change {
            n107 = event-data() -> ()  [unwired: 1 in, 5 out]
            n108 = case shown="真" "Set Zero" {
              frame False {
              }
              frame True {
                n109 = local read "Actual Positon"() -> (w312:sgl)
                n110 = local write "Set Zero Value"(w312) -> ()
              }
            }
          }
          event "Reset Zero": Value Change {
            n111 = event-data() -> ()  [unwired: 1 in, 4 out]
            n112 = local write "Set Zero Value"(sgl 0.0 ("Set Zero Value")) -> ()
          }
          event "Start": Value Change {
            n113 = event-data() -> ()  [unwired: 1 in, 5 out]
            n114 = local read "Position"() -> (→"Start Dis.":sgl)
          }
          event "End": Value Change {
            n115 = event-data() -> ()  [unwired: 1 in, 3 out]
            n116 = local read "Position"() -> (→"End Dis.":sgl)
          }
          event "Move": Value Change {
            n117 = event-data() -> ()  [unwired: 1 in, 1 out]
            n118 = invoke class="MG17Motor" method="SetJogMode"(reference=w324, error in=w323, "lChanID"=0, "lMode"=2, "lStopMode"=2) -> (reference out=w325:refnum<k7>, error out=w322:errorcluster)  [unwired: 1 in, 4 out]
            n119 = Absolute Value(x="Interval Dis.") -> (abs(x)=w329:sgl)
            n120 = Greater Than 0?(x="Interval Dis.") -> (x > 0?=w330:bool)
            n121 = case shown="假" w330 {
              tunnel: w325 -> [w345 w355]
              tunnel: [w343 w353] -> w333
              tunnel: w322 -> [w340 w350]
              tunnel: [w338 w348] -> w334
              tunnel: w329 -> [w336 w346]
              frame False {
                # "fanxiang"
                n122 = invoke class="MG17Motor" method="SetJogStepSize"(reference=w345, error in=w340, "lChanID"=0, "fStepSize"=w336) -> (reference out=w344:refnum<k7>, error out=w339:errorcluster)  [unwired: 1 in, 3 out]
                n123 = invoke class="MG17Motor" method="MoveJog"(reference=w344, error in=w339, "lChanID"=0, "lJogDir"=2) -> (reference out=w343:refnum<k7>, error out=w338:errorcluster)  [unwired: 1 in, 3 out]
              }
              frame True {
                n124 = invoke class="MG17Motor" method="SetJogStepSize"(reference=w355, error in=w350, "lChanID"=0, "fStepSize"=w346) -> (reference out=w354:refnum<k7>, error out=w349:errorcluster)  [unwired: 1 in, 3 out]
                n125 = invoke class="MG17Motor" method="MoveJog"(reference=w354, error in=w349, "lChanID"=0, "lJogDir"=0) -> (reference out=w353:refnum<k7>, error out=w348:errorcluster)  [unwired: 1 in, 3 out]
              }
            }
            n126 = property on="Z-Stack" class="Bool (严格)"(error in=w334, "Val(Sgnl)"=TRUE ("值(信号)")) -> (error out=w332:errorcluster)  [unwired: 1 in, 1 out]
          }
          event "Stop": Value Change {
            n127 = event-data() -> ()  [unwired: 1 in, 4 out]
          }
        }
        n128 = Unbundle By Name(w173) -> ("status"=w172:bool)
        n129 = Or(x=w172, y=w170) -> (x .or. y?=w171:bool)
      }
      n130 = invoke class="MG17Motor" method="StopCtrl"(reference=w169, error in=w168) -> ()  [unwired: 1 in, 3 out]
    }
  }
  n131 = xnode "Invoke Method"("FPGA VI引用输入"=w77, "错误输入"=w78) -> ("FPGA VI引用输出"=w66:refnum<k20>, "错误输出"=w67:errorcluster)
  n132 = xnode "Invoke Method"("FPGA VI引用输入"=w80, "错误输入"=w79) -> ("FPGA VI引用输出"=w63:refnum<k20>, "错误输出"=w62:errorcluster)
  n133 = xnode "Invoke Method"("FPGA VI引用输入"=w66, "错误输入"=w67) -> ("FPGA VI引用输出"=w68:refnum<k20>, "错误输出"=w69:errorcluster)
  n134 = xnode "Invoke Method"("FPGA VI引用输入"=w63, "错误输入"=w62) -> ("FPGA VI引用输出"=w61:refnum<k20>, "错误输出"=w60:errorcluster)
  n135 = xnode "Invoke Method"("FPGA VI引用输入"=w61, "错误输入"=w60) -> ("FPGA VI引用输出"=w59:refnum<k20>, "错误输出"=w58:errorcluster)  [unwired: 1 in]
  n136 = xnode "Invoke Method"("FPGA VI引用输入"=w68, "错误输入"=w69, "请求的深度"=u32 8388608) -> ("FPGA VI引用输出"=w65:refnum<k20>, "错误输出"=w64:errorcluster, "实际深度"=→"实际深度":u32)
  n137 = xnode "Invoke Method"("FPGA VI引用输入"=w65, "错误输入"=w64) -> ("FPGA VI引用输出"=w31:refnum<k20>, "错误输出"=w30:errorcluster)
  n138 = xnode "读取/写入控件"("FPGA VI引用输入"=w59, "错误输入"=w58, "Shutter"=w49, "Start Control"=w49) -> ("FPGA VI引用输出"=w51:refnum<k20>, "错误输出"=w50:errorcluster)
  n139 = xnode "Invoke Method"("FPGA VI引用输入"=w31, "错误输入"=w30) -> ("FPGA VI引用输出"=w55:refnum<k20>, "错误输出"=w54:errorcluster)  [unwired: 1 in]
  n140 = flat-sequence {
    tunnel: w5 -> [_]
    frame #0 {
      n141 = local read "Z"() -> (w359:bool)
      n142 = case shown="假" w359 {
        frame False {
          n143 = property on="Ready" class="Slide (严格)"("Label.Visible"=TRUE ("标签.可见")) -> ()  [unwired: 2 in, 2 out]
          n144 = property on="Z-Stack" class="Bool (严格)"("DisabledEnum"=T4."Enabled" ("禁用")) -> ()  [unwired: 2 in, 2 out]
          n145 = property on="LIVE" class="Bool (严格)"("DisabledEnum"=T4."Enabled" ("禁用")) -> ()  [unwired: 2 in, 2 out]
          n146 = property on="Save" class="Bool (严格)"("DisabledEnum"=T4."Enabled" ("禁用")) -> ()  [unwired: 2 in, 2 out]
          n147 = local write "Ready"(u8 10 ("Process")) -> ()
        }
        frame True {
          n148 = local write "Ready"(u8 6 ("Process")) -> ()
        }
      }
    }
  }
  n149 = while {
    tunnel: w55 -> [w373]
    tunnel: w54 -> [w372]
    tunnel: [w371] -> w19
    tunnel: [w370] -> w6
    tunnel: [w369] -> w52
    tunnel: w51 -> [w369]
    tunnel: [w368] -> w47
    tunnel: w50 -> [w368]
    stop <- w366 stop-if-true
    n150 = xnode "读取/写入控件"("FPGA VI引用输入"=w373, "错误输入"=w372) -> ("FPGA VI引用输出"=w371:refnum<k20>, "错误输出"=w370:errorcluster, "Adapter Module Initialization Done"=w366:bool)
    "Initialization Done" <- w366
    n151 = local write "Ready"(u8 3 ("Process")) -> ()
  }
  n152 = local read "Point/Pixel"() -> (w7:i32)
  n153 = property on="Point/Pixel" class="DigNum (严格)"(error in=w6, "Val(Sgnl)"=w7) -> (error out=w5:errorcluster)  [unwired: 1 in, 1 out]
  n154 = Obtain Queue(name (unnamed)="Display" ("名称（未命名）"), element data type=u16[][] []) -> (queue out=w21:refnum<queue>, error out=w22:errorcluster)  [unwired: 3 in, 1 out]
  n155 = Obtain Queue(name (unnamed)="Save" ("名称（未命名）"), element data type=u16[][] []) -> (queue out=w32:refnum<queue>, error out=w76:errorcluster)  [unwired: 3 in, 1 out]
  n156 = call "IMAQ Create"("Image Name"="Save", "Image Type"=w28) -> ("New Image"=w26:T1)  [unwired: 3 in, 1 out]
  n157 = while {
    tunnel: w19 -> [w378]
    tunnel: w5 -> [w377]
    shift-right: [w374] -> _
    shift-left: 0 ("t") -> [w375]
    stop <- w376 stop-if-true
    n158 = event shown="[2] \"Start Device\": 值改变" {
      selector: _ -> [_ _ _ _ _ _ _ _ _ _ _ _ _ _]
      dyn-events: _ -> [_ _ _ _ _ _ _ _ _ _ _ _ _ _]
      timeout: _ -> [_ _ _ _ _ _ _ _ _ _ _ _ _ _]
      tunnel: w378 -> [_ w430 _ _ _ _ _ _ _ w551 w559 w609 _ _]
      tunnel: w377 -> [_ w428 _ _ _ _ _ _ _ w550 w558 w608 _ _]
      tunnel: [_ _ _ _ _ _ _ _ _ _ _ _ _ TRUE] -> w376
      tunnel: w375 -> [w379 w417 w434 w449 w465 w486 w491 w505 w536 w549 w556 w606 w646 _]
      tunnel: [w379 w417 w434 w449 w465 w486 w491 w505 w535 w549 w556 w606 w646 u16 0 ("t")] -> w374
      event "XY RIGHT", "XY LEFT", "XY DOWN", "XY UP", "XY Home": Value Change {
        n159 = event-data() -> ()  [unwired: 1 in, 6 out]
        n160 = Build Array("XY Home", "XY UP", "XY DOWN", "XY LEFT", "XY RIGHT") -> (w385:bool[])
        n161 = Boolean Array To Number(Boolean array=w385) -> (number=w386:u32)
        n162 = case shown="16" w386 {
          tunnel: [w390 0.0 w393 w398 w403 w407] -> w388
          tunnel: [w389 0.0 w395 w399 w401 w406] -> w387
          frame 0, Default {
            n163 = local read "X Offset"() -> (w390:dbl)
            n164 = local read "Y Offset"() -> (w389:dbl)
          }
          frame 1 {
            # "Home"
          }
          frame 2 {
            # "UP"
            n165 = local read "Scale Value"() -> (w396:dbl)
            n166 = local read "X Offset"() -> (w393:dbl)
            n167 = local read "Y Offset"() -> (w394:dbl)
            n168 = Add(x=w394, y=w396) -> (x+y=w395:dbl)
          }
          frame 4 {
            # "DOWN"
            n169 = local read "Scale Value"() -> (w400:dbl)
            n170 = local read "Y Offset"() -> (w397:dbl)
            n171 = local read "X Offset"() -> (w398:dbl)
            n172 = Subtract(x=w397, y=w400) -> (x-y=w399:dbl)
          }
          frame 8 {
            # "LEFT"
            n173 = local read "Scale Value"() -> (w404:dbl)
            n174 = local read "X Offset"() -> (w402:dbl)
            n175 = local read "Y Offset"() -> (w401:dbl)
            n176 = Add(x=w402, y=w404) -> (x+y=w403:dbl)
          }
          frame 16 {
            # "RIGHT"
            n177 = local read "Scale Value"() -> (w408:dbl)
            n178 = local read "X Offset"() -> (w405:dbl)
            n179 = local read "Y Offset"() -> (w406:dbl)
            n180 = Subtract(x=w405, y=w408) -> (x-y=w407:dbl)
          }
        }
        n181 = local write "X Offset"(w388) -> ()
        n182 = local write "Y Offset"(w387) -> ()
      }
      event "Nonlinear Acq.", "Point/Pixel", "Microscope", "Wave": Value Change {
        n183 = event-data() -> ()  [unwired: 1 in, 3 out]
        n184 = local read "Wave"() -> (w411:enum16{"Triangle", "Sine", "Ramp"})
        n185 = local read "Acq. Sample Rate"() -> (w427:dbl)
        n186 = local read "X Frequency"() -> (w425:dbl)
        n187 = local read "Fill Fraction"() -> (w426:dbl)
        n188 = local read "Pixel/Line"() -> (w424:u16)
        n189 = Equal?(x=w411, y=enum16{"Triangle", "Sine", "Ramp"}."Sine") -> (x = y?=w409:bool)
        "Nonlinear Acq." <- w409
        n190 = local read "Point/Pixel"() -> (w415:i32)
        n191 = To Double Precision Float(number=w424) -> (double precision float=w423:dbl)
        n192 = call "sub_Sin Acq Point.vi"("Nonlinear Acq."=w409, "Point/Pixel"=w415, "Effecte Pixel/Line"=w423, "Fill Fraction"=w426, "Scanning Speed"=w425, "Sample Rate"=w427) -> ("Total Data Out"=→"Total Data Out":u16, "Init Data Out"=w414:u16[], "Init Data Out FXP"=w413:fxp<+,18,0>[])  [unwired: 3 in]
        "Acq.Point Array" <- w414
        "Init Data Out" <- w414
        n193 = Index Array(array=w414, index=0 ("索引")) -> (element=w418:u16)
        n194 = local write "Acq. Start"(w418) -> ()
        n195 = xnode "Invoke Method"("FPGA VI引用输入"=w430, "错误输入"=w428, "数据"=w413, "超时(ms)"=0) -> ("FPGA VI引用输出"=w422:refnum<k20>, "错误输出"=w421:errorcluster)  [unwired: 1 out]
        n196 = local read "Microscope"() -> (w412:enum16{"Miniature", "Benchtop"})
        n197 = case shown="\"Miniature\", 默认" w412 {
          frame "Miniature", Default {
            n198 = local write "Real Back Period"("Back Period") -> ()
          }
          frame "Benchtop" {
            n199 = local write "Real Back Period"(u16 1 ("Back Period")) -> ()
          }
        }
        n200 = xnode "Invoke Method"("FPGA VI引用输入"=w422, "错误输入"=w421, "数据"=w414, "超时(ms)"=0) -> ()  [unwired: 3 out]
      }
      event "Start Device": Value Change {
        n201 = event-data() -> ()  [unwired: 1 in, 6 out]
        n202 = case shown="假" "Start Device" {
          frame False {
            n203 = flat-sequence {
              frame #0 {
                n204 = local write "Mems Enable"(FALSE ("Mems Enable")) -> ()
                n205 = Wait (ms)(milliseconds to wait=u32 50 ("等待时间（毫秒）")) -> ()  [unwired: 1 out]
              }
              frame #1 {
                n206 = local write "5V"(FALSE ("5V")) -> ()
                n207 = Wait (ms)(milliseconds to wait=u32 50 ("等待时间（毫秒）")) -> ()  [unwired: 1 out]
              }
              frame #2 {
                n208 = local write "Source:Output Enabled"(FALSE ("Source:Output Enabled")) -> ()
                n209 = local write "PMT1 Enable"(FALSE ("PMT1 Enable")) -> ()
              }
            }
          }
          frame True {
            n210 = flat-sequence {
              frame #0 {
                n211 = local write "Source:Output Enabled"(TRUE ("Source:Output Enabled")) -> ()
                n212 = local write "PMT1 Enable"(TRUE ("PMT1 Enable")) -> ()
                n213 = Wait (ms)(milliseconds to wait=u32 50 ("等待时间（毫秒）")) -> ()  [unwired: 1 out]
              }
              frame #1 {
                n214 = local write "5V"(TRUE ("5V")) -> ()
                n215 = Wait (ms)(milliseconds to wait=u32 50 ("等待时间（毫秒）")) -> ()  [unwired: 1 out]
              }
              frame #2 {
                n216 = local write "Mems Enable"(TRUE ("Mems Enable")) -> ()
              }
            }
          }
        }
      }
      event "Add Phase": Value Change {
        n217 = event-data() -> ()  [unwired: 1 in, 6 out]
        n218 = local read "Scan Mode"() -> (w448:enum16{"Normal", "Line Scan", "Random Access"})
        n219 = local read "Phase Shift"() -> (w447:u32)
        n220 = case shown="\"Normal\", 默认" w448 {
          tunnel: w447 -> [w450 w451]
          frame "Random Access" {
            "Random Phase" <- w450
          }
          frame "Normal", Default {
            n221 = local read "Microscope"() -> (w459:enum16{"Miniature", "Benchtop"})
            n222 = case shown="\"Miniature\", 默认" w459 {
              tunnel: [w462 w463] -> w458
              frame "Miniature", Default {
                n223 = local read "Zoom Miniature"() -> (w462:dbl[][])
              }
              frame "Benchtop" {
                n224 = local read "Zoom Standard"() -> (w463:dbl[][])
              }
            }
            n225 = local read "ZOOM"() -> (w457:u16)
            n226 = Decrement(x=w457) -> (x-1=w455:u16)
            n227 = Index Array(array=w458, index (row)=w455) -> (element=w452:dbl[])  [unwired: 1 in]
            n228 = Insert Into Array(array=w452, index=2 ("索引"), new element=w451) -> (w454:dbl[])
            n229 = case shown="0, 默认" w457 {
              frame 0, Default {
                n230 = local read "Phase Shift"() -> (→"User Define Phase":u32)
              }
              frame 1 {
              }
            }
            n231 = Replace Array Subset(array=w458, new element=w454, index (row)=w455) -> (w456:dbl[][])  [unwired: 1 in]
            n232 = case shown="\"Miniature\", 默认" w459 {
              tunnel: w456 -> [w460 w461]
              frame "Miniature", Default {
                n233 = local write "Zoom Miniature"(w460) -> ()
              }
              frame "Benchtop" {
                n234 = local write "Zoom Standard"(w461) -> ()
              }
            }
          }
        }
      }
      event "Scan Mode", "ZOOM": Value Change {
        n235 = event-data() -> ()  [unwired: 1 in, 6 out]
        n236 = local read "Microscope"() -> (w472:enum16{"Miniature", "Benchtop"})
        n237 = case shown="\"Miniature\", 默认" w472 {
          tunnel: [w476 w477] -> w469
          frame "Miniature", Default {
            n238 = local read "Zoom Miniature"() -> (w476:dbl[][])
          }
          frame "Benchtop" {
            n239 = local read "Zoom Standard"() -> (w477:dbl[][])
          }
        }
        n240 = local read "ZOOM"() -> (w468:u16)
        n241 = case shown="0, 默认" w468 {
          selector: w468 -> [_ w481]
          tunnel: w469 -> [_ w482]
          tunnel: [w478 w480] -> w471
          frame 0, Default {
            n242 = local read "User Define Phase"() -> (w478:u32)
          }
          frame 1..10 {
            n243 = Decrement(x=w481) -> (x-1=w484:u16)
            n244 = Index Array(array=w482, index (row)=w484) -> (element=w485:dbl[])  [unwired: 1 in]
            n245 = Index Array(array=w485, index=2 ("索引")) -> (element=w479:dbl)
            n246 = To Unsigned Long Integer(number=w479) -> (unsigned 32bit integer=w480:u32)
          }
        }
        n247 = local read "Random Phase"() -> (w470:u32)
        n248 = local read "Scan Mode"() -> (w467:enum16{"Normal", "Line Scan", "Random Access"})
        n249 = case shown="\"Normal\", 默认" w467 {
          tunnel: w471 -> [w473 w474 _]
          tunnel: w470 -> [_ _ w475]
          tunnel: [w473 w474 w475] -> w466
          frame "Normal", Default {
          }
          frame "Line Scan" {
          }
          frame "Random Access" {
          }
        }
        n250 = local write "Phase Shift"(w466) -> ()
      }
      event "Set Large Scale", "Set Small Scale", "Scale": Value Change {
        n251 = event-data() -> ()  [unwired: 1 in, 6 out]
        n252 = Select(t="Set Large Scale", s="Scale", f="Set Small Scale") -> (s? t:f=→"Scale Value":dbl)
      }
      event "16-bit Display Method", "Map Max.", "Map Min.", "Max. Min.": Value Change {
        n253 = event-data() -> ()  [unwired: 1 in, 6 out]
        n254 = local read "16-bit Display Method"() -> (w492:u32)
        n255 = Unbundle("Max. Min.") -> (w495:i32, w499:i32)
        n256 = case shown="14" w492 {
          frame 0, Default {
          }
          frame 14 {
            n257 = To Double Precision Float(number="Map Max.") -> (double precision float=w502:dbl)
            n258 = To Double Precision Float(number="Map Min.") -> (double precision float=w501:dbl)
            n259 = property on="Max. Min." class="Slide (严格)"("Scale.Maximum"=w502, "Scale.Minimum"=w501) -> ()  [unwired: 2 in, 2 out]
          }
        }
        n260 = Add(x=w499, y=32768) -> (x+y=w497:i32)
        n261 = Add(x=w495, y=32768) -> (x+y=w496:i32)
        n262 = property on="Image" class="ImageControl"("16-bit Display Conversion Method"="16-bit Display Method", "16-bit Display Maximum Value"=w496, "16-bit Display Minimum Value"=w497) -> ()  [unwired: 2 in, 2 out]
      }
      event "Image": Mouse Up {
        n263 = event-data() -> ()  [unwired: 1 in, 8 out]
        n264 = disable-structure shown="禁用" {
          frame Disabled {
            n265 = local read "Microscope"() -> (w509:enum16{"Miniature", "Benchtop"})
            n266 = case shown="\"Benchtop\"" w509 {
              tunnel: [w519 w520] -> w510
              frame "Miniature", Default {
                n267 = local read "Zoom Miniature"() -> (w519:dbl[][])
              }
              frame "Benchtop" {
                n268 = local read "Zoom Standard"() -> (w520:dbl[][])
              }
            }
            n269 = local read "ZOOM"() -> (w508:u16)
            n270 = case shown="0, 默认" w508 {
              selector: w508 -> [_ w525]
              tunnel: [w521 w523] -> w506
              tunnel: [w522 w524] -> w507
              tunnel: w510 -> [_ w526]
              frame 0, Default {
                n271 = local read "X Amplitude"() -> (w522:dbl)
                n272 = local read "Y Amplitude"() -> (w521:dbl)
              }
              frame 1..10 {
                n273 = Decrement(x=w525) -> (x-1=w529:u16)
                n274 = Index Array(array=w526, index (row)=w529) -> (element=w530:dbl[])  [unwired: 1 in]
                n275 = Index Array(array=w530, index #1=0 ("索引"), index #2=1 ("索引")) -> (element #1=w524:dbl, element #2=w523:dbl)  [unwired: 1 in, 1 out]
              }
            }
            n276 = property on="Image" class="ImageControl"() -> ("ROI"=w518:T5)  [unwired: 2 in, 2 out]
            n277 = local read "Pixel/Line"() -> (w515:u16)
            n278 = local read "Line"() -> (w514:u32)
            n279 = Unbundle By Name(w518) -> ("Global Rectangle"=w517:i32[])
            n280 = call "sub_new x y amplitude.vi"("Global Rectangle"=w517, "Line"=w514, "Pixel/Line"=w515, "y amp."=w506, "x amp."=w507) -> ("y offset new"=→"y offset new":i16, "x offset new"=→"x offset new":i16, "y amp. new"=→"y amp. new":dbl, "x amp. new"=→"x amp. new":dbl)  [unwired: 3 in]
          }
          frame Enabled {
          }
        }
      }
      event "Add Random Access", "Clear Array": Value Change {
        n281 = event-data() -> ()  [unwired: 1 in, 6 out]
        n282 = case shown="真" "Add Random Access" {
          tunnel: w536 -> [w539 w543]
          tunnel: [w539 w544] -> w533
          frame False {
          }
          frame True {
            n283 = local read "x amp. new"() -> (w548:dbl)
            n284 = local read "y amp. new"() -> (w547:dbl)
            n285 = local read "x offset new"() -> (w546:i16)
            n286 = local read "y offset new"() -> (w545:i16)
            n287 = call "sub_new amplitude to array.vi"("Index Row"=w543, "All Random Array In"="All Random Array", "y offset new"=w545, "x offset new"=w546, "y amp. new"=w547, "x amp. new"=w548) -> ("All Random Array Out"=w541:fxp<+/-,32,16>[][])  [unwired: 4 in, 1 out]
            n288 = Increment(x=w543) -> (x+1=w544:i32)
            n289 = local write "All Random Array"(w541) -> ()
            n290 = call "sub_2D Array to 1D.vi"("2D Array"=w541) -> ("Random 1D Array"=w540:fxp<+/-,32,16>[])
            n291 = local write "Random 1D Array"(w540) -> ()
          }
        }
        n292 = case shown="真" "Clear Array" {
          frame False {
          }
          frame True {
            n293 = local write "Random 1D Array"(fxp<+/-,32,16>[] [0.0, 0.0, 0.0, 0.0, 0.0, 0.0, 0.0, 0.0, 0.0, 0.0, 0.0, 0.0, 0.0, 0.0, 0.0, 0.0, 0.0, 0.0, 0.0, 0.0, 0.0, 0.0, 0.0, 0.0, 0.0, 0.0, 0.0, 0.0, 0.0, 0.0, 0.0, 0.0, 0.0, 0.0, 0.0, 0.0, 0.0, 0.0, 0.0, 0.0, 0.0, 0.0, 0.0, 0.0, 0.0, 0.0, 0.0, 0.0, 0.0, 0.0, 0.0, 0.0, 0.0, 0.0, 0.0, 0.0, 0.0, 0.0, 0.0, 0.0, 0.0, 0.0, 0.0, 0.0, 0.0, 0.0, 0.0, 0.0, 0.0, 0.0, 0.0, 0.0, 0.0, 0.0, 0.0, 0.0, 0.0, 0.0, 0.0, 0.0, 0.0, 0.0, 0.0, 0.0, 0.0, 0.0, 0.0, 0.0, 0.0, 0.0, 0.0, 0.0, 0.0, 0.0, 0.0, 0.0, 0.0, 0.0, 0.0, 0.0, 0.0, 0.0, 0.0, 0.0, 0.0, 0.0, 0.0, 0.0, 0.0, 0.0, 0.0, 0.0, 0.0, 0.0, 0.0, 0.0, 0.0, 0.0, 0.0, 0.0, 0.0, 0.0, 0.0, 0.0, 0.0, 0.0, 0.0, 0.0, 0.0, 0.0, 0.0, 0.0, 0.0, 0.0, 0.0, 0.0, 0.0, 0.0, 0.0, 0.0, 0.0, 0.0, 0.0, 0.0, 0.0, 0.0, 0.0, 0.0, 0.0, 0.0, 0.0, 0.0, 0.0, 0.0, 0.0, 0.0, 0.0, 0.0, 0.0, 0.0, 0.0, 0.0, 0.0, 0.0, 0.0, 0.0, 0.0, 0.0, 0.0, 0.0, 0.0, 0.0, 0.0, 0.0, 0.0, 0.0, 0.0, 0.0, 0.0, 0.0, 0.0, 0.0, 0.0, 0.0, 0.0, 0.0, 0.0, 0.0, 0.0, 0.0, 0.0, 0.0, 0.0, 0.0, 0.0, 0.0, 0.0, 0.0, 0.0, 0.0] ("Random 1D Array")) -> ()
            n294 = local write "All Random Array"(fxp<+/-,32,16>[][] [] ("All Random Array")) -> ()
          }
        }
        n295 = Select(t=0, s="Clear Array", f=w533) -> (s? t:f=w535:i32)
      }
      event "Apply": Value Change {
        n296 = event-data() -> ()  [unwired: 1 in, 6 out]
        n297 = xnode "读取/写入控件"("FPGA VI引用输入"=w551, "错误输入"=w550, "Adapter Module User Command"="Adapter Module User Command", "Adapter Module User Data 0"="Adapter Module User Data 0", "Adapter Module User Data 1"="Adapter Module User Data 1", "Adapter Module Do User Command Commit"="Apply") -> ()  [unwired: 2 out]
      }
      event "Gain": Value Change {
        n298 = event-data() -> ()  [unwired: 1 in, 6 out]
        n299 = local read "Microscope"() -> (w557:enum16{"Miniature", "Benchtop"})
        n300 = case shown="\"0dB\", 默认" "Gain" {
          tunnel: w559 -> [w563 w578 w593]
          tunnel: w558 -> [w562 w577 w592]
          tunnel: w557 -> [w561 w576 w591]
          frame "0dB", Default {
            n301 = case shown="\"Miniature\", 默认" w561 {
              tunnel: w563 -> [w569 w571]
              tunnel: w562 -> [w568 w570]
              frame "Miniature", Default {
                n302 = xnode "读取/写入控件"("FPGA VI引用输入"=w569, "错误输入"=w568, "Adapter Module User Command"=u8 2, "Adapter Module User Data 0"=u8 0, "Adapter Module User Data 1"=u8 0, "Adapter Module Do User Command Commit"=TRUE) -> ()  [unwired: 2 out]
              }
              frame "Benchtop" {
                n303 = xnode "读取/写入控件"("FPGA VI引用输入"=w571, "错误输入"=w570, "Adapter Module User Command"=u8 2, "Adapter Module User Data 0"=u8 1, "Adapter Module User Data 1"=u8 0, "Adapter Module Do User Command Commit"=TRUE) -> ()  [unwired: 2 out]
              }
            }
          }
          frame "6dB" {
            n304 = case shown="\"Benchtop\"" w576 {
              tunnel: w578 -> [w584 w586]
              tunnel: w577 -> [w583 w585]
              frame "Miniature", Default {
                n305 = xnode "读取/写入控件"("FPGA VI引用输入"=w584, "错误输入"=w583, "Adapter Module User Command"=u8 2, "Adapter Module User Data 0"=u8 0, "Adapter Module User Data 1"=u8 1, "Adapter Module Do User Command Commit"=TRUE) -> ()  [unwired: 2 out]
              }
              frame "Benchtop" {
                n306 = xnode "读取/写入控件"("FPGA VI引用输入"=w586, "错误输入"=w585, "Adapter Module User Command"=u8 2, "Adapter Module User Data 0"=u8 1, "Adapter Module User Data 1"=u8 1, "Adapter Module Do User Command Commit"=TRUE) -> ()  [unwired: 2 out]
              }
            }
          }
          frame "12dB" {
            n307 = case shown="\"Miniature\", 默认" w591 {
              tunnel: w593 -> [w595 w605]
              tunnel: w592 -> [w594 w604]
              frame "Miniature", Default {
                n308 = xnode "读取/写入控件"("FPGA VI引用输入"=w595, "错误输入"=w594, "Adapter Module User Command"=u8 2, "Adapter Module User Data 0"=u8 0, "Adapter Module User Data 1"=u8 2, "Adapter Module Do User Command Commit"=TRUE) -> ()  [unwired: 2 out]
              }
              frame "Benchtop" {
                n309 = xnode "读取/写入控件"("FPGA VI引用输入"=w605, "错误输入"=w604, "Adapter Module User Command"=u8 2, "Adapter Module User Data 0"=u8 1, "Adapter Module User Data 1"=u8 2, "Adapter Module Do User Command Commit"=TRUE) -> ()  [unwired: 2 out]
              }
            }
          }
        }
      }
      event "Coulple": Value Change {
        n310 = event-data() -> ()  [unwired: 1 in, 6 out]
        n311 = local read "Microscope"() -> (w607:enum16{"Miniature", "Benchtop"})
        n312 = case shown="\"AC\", 默认" "Coulple" {
          tunnel: w609 -> [w613 w628]
          tunnel: w608 -> [w612 w627]
          tunnel: w607 -> [w611 w626]
          frame "AC", Default {
            n313 = case shown="\"Benchtop\"" w611 {
              tunnel: w613 -> [w615 w621]
              tunnel: w612 -> [w614 w620]
              frame "Miniature", Default {
                n314 = xnode "读取/写入控件"("FPGA VI引用输入"=w615, "错误输入"=w614, "Adapter Module User Command"=u8 3, "Adapter Module User Data 0"=u8 0, "Adapter Module User Data 1"=u8 0, "Adapter Module Do User Command Commit"=TRUE) -> ()  [unwired: 2 out]
              }
              frame "Benchtop" {
                n315 = xnode "读取/写入控件"("FPGA VI引用输入"=w621, "错误输入"=w620, "Adapter Module User Command"=u8 3, "Adapter Module User Data 0"=u8 1, "Adapter Module User Data 1"=u8 0, "Adapter Module Do User Command Commit"=TRUE) -> ()  [unwired: 2 out]
              }
            }
          }
          frame "DC" {
            n316 = case shown="\"Benchtop\"" w626 {
              tunnel: w628 -> [w630 w636]
              tunnel: w627 -> [w629 w635]
              frame "Miniature", Default {
                n317 = xnode "读取/写入控件"("FPGA VI引用输入"=w630, "错误输入"=w629, "Adapter Module User Command"=u8 3, "Adapter Module User Data 0"=u8 0, "Adapter Module User Data 1"=u8 1, "Adapter Module Do User Command Commit"=TRUE) -> ()  [unwired: 2 out]
              }
              frame "Benchtop" {
                n318 = xnode "读取/写入控件"("FPGA VI引用输入"=w636, "错误输入"=w635, "Adapter Module User Command"=u8 3, "Adapter Module User Data 0"=u8 1, "Adapter Module User Data 1"=u8 1, "Adapter Module Do User Command Commit"=TRUE) -> ()  [unwired: 2 out]
              }
            }
          }
        }
      }
      event "Frames/Slice", "Slices": Value Change {
        n319 = event-data() -> ()  [unwired: 1 in, 6 out]
        n320 = local read "Start Dis."() -> (w644:sgl)
        n321 = local read "End Dis."() -> (w645:sgl)
        n322 = Subtract(x=w645, y=w644) -> (x-y=w643:sgl)
        n323 = Divide(x=w643, y="Slices") -> (x/y=w641:sgl)
        n324 = local write "Interval Dis."(w641) -> ()
      }
      event "Stop": Value Change {
        n325 = event-data() -> ()  [unwired: 1 in, 6 out]
      }
    }
  }
  n326 = while {
    tunnel: [w654] -> w57
    tunnel: [w653] -> w56
    tunnel: w52 -> [w652]
    tunnel: w47 -> [w651]
    stop <- w649 stop-if-true
    n327 = event shown="[0] 超时" {
      selector: _ -> [_ _]
      dyn-events: _ -> [_ _]
      timeout: 1 -> [_ _]
      tunnel: [w691 w773] -> w654
      tunnel: [w690 w772] -> w653
      tunnel: w652 -> [w693 w775]
      tunnel: w651 -> [w692 w774]
      tunnel: [_ TRUE ("FPGA Stop")] -> w649
      event Timeout {
        n328 = event-data() -> ()  [unwired: 1 in, 3 out]
        n329 = local read "Pulse Number"() -> (w673:enum16{"SP", "DP"})
        n330 = local read "Acq. Sample Rate"() -> (w663:dbl)
        n331 = Equal?(x=w673, y=enum16{"SP", "DP"}."SP") -> (x = y?=w671:bool)
        n332 = local read "Microscope"() -> (w714:enum16{"Miniature", "Benchtop"})
        n333 = case shown="\"Benchtop\"" w714 {
          tunnel: ["Zoom Miniature" "Zoom Standard"] -> w713
          frame "Miniature", Default {
          }
          frame "Benchtop" {
          }
        }
        n334 = local read "Total Data Out"() -> (w667:u16)
        n335 = Select(t=1.0, s=w671, f=2.0 ("t")) -> (s? t:f=w670:dbl)
        n336 = local read "Wave"() -> (w674:enum16{"Triangle", "Sine", "Ramp"})
        n337 = call "sub_MEMS Value to Frequency.vi"("MEMS FAST"="MEMS FAST") -> ("Ticks"=w724:u32)  [unwired: 10 in]
        n338 = call "sub_MEMS Value to Frequency.vi"("MEMS FAST"="MEMS SLOW") -> ("Ticks"=w725:u32)  [unwired: 10 in]
        n339 = case shown="0, 默认" "ZOOM" {
          selector: "ZOOM" -> [_ w765]
          tunnel: ["Y Amplitude" w763] -> w711
          tunnel: ["X Amplitude" w764] -> w716
          tunnel: w713 -> [_ w766]
          frame 0, Default {
          }
          frame 1..10 {
            n340 = Decrement(x=w765) -> (x-1=w769:u16)
            n341 = Index Array(array=w766, index (row)=w769) -> (element=w770:dbl[])  [unwired: 1 in]
            n342 = Index Array(array=w770, index #1=0 ("索引"), index #2=1 ("索引")) -> (element #1=w764:dbl, element #2=w763:dbl)  [unwired: 1 in, 1 out]
          }
        }
        n343 = local read "Line"() -> (w729:u32)
        n344 = Multiply(x="X Frequency", y=w670) -> (x*y=w731:dbl)
        n345 = Divide(x=w731, y=w729) -> (x/y=→"Frame Rate":dbl)
        n346 = call "sub_HOSTTOFPGA Voltage.vi"("Input"="Y Offset") -> ("Output"=w701:i16)
        n347 = call "sub_HOSTTOFPGA Voltage.vi"("Input"="X Offset") -> ("Output"=w666:i16)
        n348 = call "sub_HOSTTOFPGA Voltage.vi"("Input"="Laser Intensity") -> ("Output"=w698:i16)
        n349 = call "sub_HOSTTOFPGA Voltage.vi"("Input"="PMT1 Sensitivity") -> ("Output"=w705:i16)
        n350 = call "sub_HOSTTOFPGA Voltage.vi"("Input"="PMT2 Sensitivity") -> ("Output"=w684:i16)
        n351 = To Word Integer(number=w705) -> (16bit integer=w752:i16)
        n352 = case shown="\"Line Scan\"" "Scan Mode" {
          tunnel: [w756 0.0 ("数值输入控件") w758] -> w717
          tunnel: w711 -> [w756 _ w758]
          frame "Normal", Default {
          }
          frame "Line Scan" {
          }
          frame "Random Access" {
          }
        }
        n353 = To Word Integer(number=w684) -> (16bit integer=w682:i16)
        n354 = To Word Integer(number=w698) -> (16bit integer=w699:i16)
        n355 = local read "Acq. Sample Rate"() -> (w664:dbl)
        n356 = call "sub_XY Amplitude Regular.vi"("Y Amplitude"=w717, "X Amplitude"=w716) -> ("Y Amplitude Out"=w719:fxp<+,16,0>, "X Amplitude Out"=w718:fxp<+,16,0>)  [unwired: 8 in]
        n357 = local read "Wave"() -> (w678:enum16{"Triangle", "Sine", "Ramp"})
        n358 = case shown="\"SP\"" "Pulse Number" {
          tunnel: [enum16{"Single Pulse", "Two Pulse"}."Two Pulse" ("Pulse Number") enum16{"Single Pulse", "Two Pulse"}."Single Pulse" ("Pulse Number")] -> w677
          frame "DP" {
          }
          frame "SP" {
          }
        }
        n359 = call "sub_calculate value.vi"("Pixel/Line"="Pixel/Line", "Fill Fraction"="Fill Fraction", "Wave"=w678, "X Frequency"="X Frequency", "Acq. Sample Rate"=w664) -> ("Pixel Dwell"=→"Pixel Dwell":dbl, "Point/Pixel"=w661:i32)  [unwired: 5 in]
        "Point/Pixel" <- w661
        n360 = feedback #1() -> (w656:u32)  [unwired: 1 in]
        n361 = call "sub_calculate xyfrequency.vi"("Total Data Out"=w667, "Line"="Line", "Actual Output Ticks"=w656, "Actual DDS Ticks"=w656, "X Frequency"="X Frequency", "Acq. Sample Rate"=w663, "Fill Fraction"="Fill Fraction", "Back Period"="Real Back Period", "Wave"=w674) -> ("Actual DDS Sample Freq"=w697:u32, "Y Ramp Step"=w665:fxp<+/-,24,16>, "Line Out"=w695:u32, "Acq. Latch Time"=w700:u32, "Y Step"=w694:fxp<+/-,24,16>)  [unwired: 2 in]
        "Actual DDS Sample Freq" <- w697
        n362 = xnode "读取/写入控件"("FPGA VI引用输入"=w693, "错误输入"=w692, "Phase Increse"=w697, "Y Ramp Step"=w665, "Line"=w695, "Y Step"=w694, "Latch Time"=w700, "Back Period"="Real Back Period", "Laser Intensity"=w699, "X Offset"=w666, "Y Offset"=w701, "MEMS FAST"=w724, "MEMS SLOW"=w725, "PMT Sensitivity"=w752, "PMT2 Sensitivity"=w682, "X Amplitude"=w718, "Y Amplitude"=w719, "Syn. Latch Time"=u32 4 ("Latch Time"), "Pulse Number"=w677) -> ("FPGA VI引用输出"=w702:refnum<k20>, "错误输出"=w703:errorcluster, "Actual DDS Ticks"=w696:u32)
        "Actual DDS Ticks" <- w696
        n363 = feedback-in #1(w696) -> ()
        n364 = call "sub_HOSTTOFPGA Voltage.vi"("Input"="Stimulate Value") -> ("Output"=w732:i16)
        n365 = Increment(x="Frames Befor Stimulate") -> (x+1=w737:u32)
        n366 = Multiply(x="Stimulate Time", y=u32 500) -> (x*y=w739:u32)
        n367 = To Word Integer(number=w732) -> (16bit integer=w741:i16)
        n368 = xnode "读取/写入控件"("FPGA VI引用输入"=w702, "错误输入"=w703, "DDS Ticks"="DDS Ticks", "Phase Shift"="Phase Shift", "Microscope"="Microscope", "Point"="Point", "PMT1 Enable"="PMT1 Enable", "PMT2 Enable"="PMT2 Switch", "Frames Befor Stimulate"=w737, "Stimulate Interval"="Stimulate Interval", "Stimulate Time"=w739, "Stimulate Enable"="Stimulate Enable", "Vision Stimulate Value"=w741, "Wave"="Wave", "MEMS Enable"="Mems Enable", "OUTPUT Value Ticks"="OUTPUT Value Ticks", "PMT Shutter Pow."="PMT Shutter Pow.") -> ("FPGA VI引用输出"=w691:refnum<k20>, "错误输出"=w690:errorcluster, "Actual Laser Intensity"=w721:i16, "Frame Number"=w750:u32, "Stmulate Interval Dis."=→"Stimulate Time Dis.":u32, "Shock Detection"=→"Overload Dis.":bool, "Actual OUTPUT Value Ticks"=→"Actual OUTPUT Value Ticks":u32)
        n369 = call "值已改变(I32).vi"("输入数据"=w661) -> ("已更改"=w662:bool)  [unwired: 3 in]
        n370 = case shown="真" w662 {
          tunnel: w661 -> [_ w753]
          frame False {
          }
          frame True {
            n371 = property on="Point/Pixel" class="DigNum (严格)"("Val(Sgnl)"=w753) -> ()  [unwired: 2 in, 2 out]
          }
        }
        n372 = local read "Stimulate Interval"() -> (w749:u32)
        n373 = call "sub_FPGATOHOST Voltage.vi"("Input"=w721) -> ("Output"=→"Actual Laser Intensity":dbl)
        n374 = local read "Frame Rate"() -> (w748:dbl)
        n375 = Decrement(x=w750) -> (x-1=w745:u32)
        "Frame Number" <- w745
        n376 = To Double Precision Float(number=w745) -> (double precision float=w744:dbl)
        n377 = Reciprocal(x=w748) -> (1/x=w743:dbl)
        n378 = To Double Precision Float(number=w749) -> (double precision float=w746:dbl)
        n379 = Multiply(x=w744, y=w743) -> (x*y=→"Frame Befor Time":dbl)
        n380 = Multiply(x=w746, y=w743) -> (x*y=→"Stimulate Interval Time":dbl)
      }
      event "Stop": Value Change {
        n381 = event-data() -> ()  [unwired: 1 in, 3 out]
        n382 = xnode "读取/写入控件"("FPGA VI引用输入"=w775, "错误输入"=w774, "FPGA Stop"=TRUE) -> ("FPGA VI引用输出"=w777:refnum<k20>, "错误输出"=w778:errorcluster)
        n383 = xnode "Invoke Method"("FPGA VI引用输入"=w777, "错误输入"=w778) -> ("FPGA VI引用输出"=w773:refnum<k20>, "错误输出"=w772:errorcluster)
      }
    }
  }
  n384 = while {
    tunnel: w32 -> [w787]
    shift-right: [w783] -> _
    shift-left: u16 0 -> [w784]
    tunnel: w26 -> [w782]
    shift-right: [w780] -> _
    shift-left: u16 0 -> [w781]
    stop <- w779 stop-if-true
    n385 = Dequeue Element(queue=w787) -> (element=w785:u16[][], error out=w786:errorcluster)  [unwired: 2 in, 2 out]
    n386 = case shown="无错误" w786 {
      tunnel: w785 -> [w791 _]
      tunnel: w784 -> [w804 w860]
      tunnel: [w803 w860] -> w783
      tunnel: w782 -> [w801 _]
      tunnel: w781 -> [w794 w859]
      tunnel: [w793 w859] -> w780
      tunnel: [FALSE TRUE] -> w779
      frame No Error {
        # "高"
        # "低"
        n387 = local read "Pulse Number"() -> (w789:enum16{"SP", "DP"})
        n388 = call "sub_数组奇数行转置.vi"("Pulse Number"=w789, "Input"=w791) -> ("output"=w790:u16[][])
        n389 = local read "Z-Stack"() -> (w799:bool)
        n390 = Subtract(x=u16 65535, y=w790) -> (x-y=w788:u16[][])
        n391 = Build Array("Save", w799) -> (w798:bool[])
        n392 = Boolean Array To Number(Boolean array=w798) -> (number=w797:u32)
        n393 = case shown="1" w797 {
          tunnel: w804 -> [w806 w822 w832 w856]
          tunnel: [u16 0 w821 w835 u16 0] -> w803
          tunnel: w801 -> [_ w820 w840 _]
          tunnel: w788 -> [_ w819 w838 _]
          tunnel: "Path" -> [_ w818 w837 _]
          tunnel: [w806 w817 w828 w856] -> w795
          tunnel: w794 -> [_ _ w831 _]
          tunnel: [u16 0 ("t") u16 0 ("t") w834 u16 0] -> w793
          frame 0, Default {
          }
          frame 1 {
            # "Save"
            n394 = call "IMAQ ArrayToImage"("Image Pixels (U16)"=w819, "Image"=w820) -> ("Image Out"=w809:T1)  [unwired: 8 in, 1 out]
            n395 = Number To Decimal String(number=w822) -> (decimal integer string=w814:string)  [unwired: 1 in]
            n396 = Increment(x=w822) -> (x+1=w817:u16)
            n397 = Concatenate Strings("File Name", w814, ".tif" ("字符串")) -> (w815:string)
            n398 = Greater Or Equal?(x=w817, y="Save Frames") -> (x >= y?=w810:bool)
            n399 = case shown="真" w810 {
              tunnel: [w823 u16 0] -> w821
              tunnel: w817 -> [w823 _]
              frame False {
              }
              frame True {
                n400 = property on="Save" class="Bool (严格)"("Val(Sgnl)"=FALSE ("Save")) -> ()  [unwired: 2 in, 2 out]
              }
            }
            n401 = Build Path(base path=w818, name or relative path=w815) -> (appended path=w812:path)
            n402 = call-poly "IMAQ Write File 2"("File Path"=w812, "Image"=w809) -> ()  [unwired: 8 in, 2 out]
          }
          frame 2 {
            # "Z-Stack"
            n403 = local read "Frames/Slice"() -> (w830:u16)
            n404 = call "IMAQ ArrayToImage"("Image Pixels (U16)"=w838, "Image"=w840) -> ("Image Out"=w839:T1)  [unwired: 8 in, 1 out]
            n405 = Multiply(x=w831, y=w830) -> (x*y=w833:u16)
            n406 = Add(x=w833, y=w832) -> (x+y=w829:u16)
            n407 = Increment(x=w832) -> (x+1=w836:u16)
            n408 = Number To Decimal String(number=w829) -> (decimal integer string=w843:string)  [unwired: 1 in]
            n409 = local read "File Name"() -> (w826:string)
            n410 = Greater Or Equal?(x=w836, y=w830) -> (x >= y?=w827:bool)
            n411 = case shown="真" w827 {
              tunnel: w836 -> [w846 _]
              tunnel: w831 -> [w845 w851]
              tunnel: [w846 u16 0 ("t")] -> w835
              tunnel: [w845 w849] -> w834
              frame False {
              }
              frame True {
                n412 = local read "Slices"() -> (w847:u16)
                n413 = Increment(x=w851) -> (x+1=w848:u16)
                n414 = property on="Z-Stack" class="Bool (严格)"("Val(Sgnl)"=FALSE ("Save")) -> ()  [unwired: 2 in, 2 out]
                n415 = Greater Or Equal?(x=w848, y=w847) -> (x >= y?=w852:bool)
                n416 = Select(t=u16 0, s=w852, f=w848) -> (s? t:f=w849:u16)
              }
            }
            n417 = Concatenate Strings(w826, w843, ".tif" ("字符串")) -> (w844:string)
            n418 = Increment(x=w829) -> (x+1=w828:u16)
            n419 = Build Path(base path=w837, name or relative path=w844) -> (appended path=w841:path)
            n420 = call-poly "IMAQ Write File 2"("File Path"=w841, "Image"=w839) -> ()  [unwired: 8 in, 2 out]
          }
          frame 3 {
          }
        }
        "Save Frames Dis." <- w795
      }
      frame Error {
      }
    }
  }
  n421 = while {
    tunnel: w19 -> [w876]
    tunnel: w5 -> [w875]
    tunnel: [w874] -> w72
    tunnel: [w873] -> w71
    tunnel: w32 -> [w872]
    tunnel: w76 -> [w871]
    tunnel: [w870] -> w73
    tunnel: w52 -> [w867]
    tunnel: w47 -> [w866]
    border: u32 0 -> [_]
    shift-right: [w864] -> _
    shift-left: u16 0 -> [w865]
    tunnel: w21 -> [w863]
    tunnel: w22 -> [w862]
    tunnel: [w861] -> w20
    stop <- w869 stop-if-true
    # "Z-stack"
    n422 = event shown="[2] \"Z-Stack\": 值改变" {
      selector: _ -> [_ _ _ _ _]
      dyn-events: _ -> [_ _ _ _ _]
      timeout: 1 -> [_ _ _ _ _]
      tunnel: w876 -> [w892 w979 w1084 w1224 w1251]
      tunnel: w875 -> [w891 w978 w1083 w1223 w1250]
      tunnel: [w898 w977 w1082 w1221 w1253] -> w874
      tunnel: [w894 w971 w1076 w1220 w1252] -> w873
      tunnel: w872 -> [w897 _ _ _ _]
      tunnel: w871 -> [w896 w976 w1081 w1218 w1248]
      tunnel: [w895 w976 w1081 w1218 w1248] -> w870
      tunnel: [_ _ _ _ TRUE] -> w869
      tunnel: w867 -> [_ w975 w1080 _ _]
      tunnel: w866 -> [_ w974 w1079 _ _]
      tunnel: w865 -> [w893 _ w1074 w1219 w1247]
      tunnel: [w893 u16 0 w1073 w1219 w1247] -> w864
      tunnel: w863 -> [w889 _ _ _ _]
      tunnel: w862 -> [w888 w968 w1072 w1211 w1246]
      tunnel: [w887 w968 w1072 w1211 w1246] -> w861
      event Timeout {
        n423 = event-data() -> ()  [unwired: 1 in, 3 out]
        n424 = local read "Microscope"() -> (w877:enum16{"Miniature", "Benchtop"})
        n425 = local read "Pixel/Line"() -> (w881:u16)
        n426 = local read "Line"() -> (w880:u32)
        n427 = Reciprocal(x="Acq. Start") -> (1/x=w885:dbl)
        n428 = To Fixed-Point(fixed-point type=fxp<+,18,0> 0.0, number=w885) -> (fixed-point=w884:fxp<+,18,0>)
        n429 = case shown="真" "Focus Flag" {
          tunnel: w892 -> [w906 w923]
          tunnel: w891 -> [w905 w922]
          tunnel: [w904 w930] -> w898
          tunnel: w897 -> [_ w933]
          tunnel: w896 -> [w912 w932]
          tunnel: [w912 w931] -> w895
          tunnel: [w903 w929] -> w894
          tunnel: w881 -> [_ w924]
          tunnel: w880 -> [_ w925]
          tunnel: w889 -> [_ w928]
          tunnel: w888 -> [w901 w927]
          tunnel: [w901 w926] -> w887
          frame False {
            (unwired) u32 0 ("剩余元素")
            n430 = xnode "Invoke Method"("FPGA VI引用输入"=w906, "错误输入"=w905, "元素数量"=u32 0, "超时(ms)"=0) -> ("FPGA VI引用输出"=w908:refnum<k20>, "错误输出"=w909:errorcluster, "剩余元素"=w900:u32)  [unwired: 1 out]
            n431 = Not Equal To 0?(x=w900) -> (x != 0?=w902:bool)
            n432 = local write "Rolling Queue Flag"(TRUE ("Rolling Queue Flag")) -> ()
            n433 = xnode "Invoke Method"("FPGA VI引用输入"=w908, "错误输入"=w909, "元素数量"=w900, "超时(ms)"=0) -> ("FPGA VI引用输出"=w904:refnum<k20>, "错误输出"=w903:errorcluster)  [unwired: 2 out]
            n434 = case shown="真" w902 {
              frame False {
              }
              frame True {
                n435 = feedback #2() -> (w913:u32)
                n436 = Increment(x=w913) -> (x+1=w914:u32)
                "Test Point" <- w914
                n437 = feedback-in #2(w914) -> ()
              }
            }
          }
          frame True {
            n438 = xnode "Invoke Method"("FPGA VI引用输入"=w923, "错误输入"=w922, "元素数量"=u32 0, "超时(ms)"=0) -> ("FPGA VI引用输出"=w921:refnum<k20>, "错误输出"=w920:errorcluster, "剩余元素"=w919:u32)  [unwired: 1 out]
            n439 = Multiply(x=w924, y=w925) -> (x*y=w918:u32)
            n440 = Greater Or Equal?(x=w919, y=w918) -> (x >= y?=w917:bool)
            n441 = case shown="真" w917 {
              tunnel: w933 -> [_ w957]
              tunnel: w932 -> [w935 w956]
              tunnel: [w935 w955] -> w931
              tunnel: [w937 w954] -> w930
              tunnel: [w936 w953] -> w929
              tunnel: w920 -> [w936 w952]
              tunnel: w921 -> [w937 w951]
              tunnel: w925 -> [_ w942]
              tunnel: w924 -> [_ w941]
              tunnel: w928 -> [_ w950]
              tunnel: w927 -> [w934 w949]
              tunnel: [w934 w948] -> w926
              tunnel: w918 -> [_ w947]
              frame False {
              }
              frame True {
                n442 = xnode "Invoke Method"("FPGA VI引用输入"=w951, "错误输入"=w952, "元素数量"=w947, "超时(ms)"=0) -> ("FPGA VI引用输出"=w954:refnum<k20>, "错误输出"=w953:errorcluster, "数据"=w938:fxp<+,33,17>[])  [unwired: 1 out]
                n443 = Reshape Array(w938, w942, w941) -> (w939:fxp<+,33,17>[][])
                n444 = To Unsigned Word Integer(number=w939) -> (unsigned 16bit integer=w940:u16[][])
                n445 = local read "Z-Stack"() -> (w945:bool)
                n446 = local read "Save"() -> (w944:bool)
                n447 = Enqueue Element(queue=w950, element=w940, error in (no error)=w949) -> (error out=w948:errorcluster)  [unwired: 1 in, 2 out]
                n448 = Or(x=w945, y=w944) -> (x .or. y?=w943:bool)
                n449 = case shown="真" w943 {
                  tunnel: w957 -> [_ w962]
                  tunnel: w956 -> [w958 w961]
                  tunnel: [w958 w960] -> w955
                  tunnel: w940 -> [_ w959]
                  frame False {
                  }
                  frame True {
                    n450 = Enqueue Element(queue=w962, element=w959, error in (no error)=w961) -> (error out=w960:errorcluster)  [unwired: 1 in, 2 out]
                  }
                }
              }
            }
          }
        }
        n451 = xnode "读取/写入控件"("FPGA VI引用输入"=w892, "Pixel/Line"=w881, "Line"=w880, "Microscope"=w877, "Acq.Start FXP"=w884, "Acq.Start"="Acq. Start", "Divide"="Divide") -> ("Acq. Point Dis."=→"Acq. Point Dis.":u16)  [unwired: 1 in, 2 out]
        n452 = call "sub_Acquisition Rate.vi"("Divide"="Divide") -> ("采样率"=→"Acq. Sample Rate":dbl)
      }
      event "LIVE", "Save": Value Change {
        (unwired) 0
        (unwired) u16 0
        # "高"
        # "低"
        n453 = event-data() -> ()  [unwired: 1 in, 6 out]
        n454 = local read "Save"() -> (w964:bool)
        n455 = global write "Save picture camera.vi" "Save Picture Camera"(w964) -> ()
        n456 = Compound Arithmetic op=OR ("复合运算")("LIVE", w964) -> (w966:bool)
        n457 = Build Array(w964, "LIVE") -> (w970:bool[])
        n458 = Boolean Array To Number(Boolean array=w970) -> (number=w969:u32)
        n459 = case shown="0, 默认" w969 {
          frame 1 {
            # "SAVE 1"
            # "LIVE 0"
            n460 = property on="LIVE" class="Bool (严格)"("DisabledEnum"=T4."Disabled and Grayed Out" ("禁用")) -> ()  [unwired: 2 in, 2 out]
            n461 = property on="Z-Stack" class="Bool (严格)"("DisabledEnum"=T4."Disabled and Grayed Out" ("禁用")) -> ()  [unwired: 2 in, 2 out]
          }
          frame 2 {
            # "SAVE 0"
            # "LIVE 1"
            n462 = property on="Save" class="Bool (严格)"("DisabledEnum"=T4."Disabled and Grayed Out" ("禁用")) -> ()  [unwired: 2 in, 2 out]
            n463 = property on="Z-Stack" class="Bool (严格)"("DisabledEnum"=T4."Disabled and Grayed Out" ("禁用")) -> ()  [unwired: 2 in, 2 out]
          }
          frame 0, Default {
            # "SAVE 0"
            # "LIVE 0"
            n464 = property on="Save" class="Bool (严格)"("DisabledEnum"=T4."Enabled" ("禁用")) -> ()  [unwired: 2 in, 2 out]
            n465 = property on="LIVE" class="Bool (严格)"("DisabledEnum"=T4."Enabled" ("禁用")) -> ()  [unwired: 2 in, 2 out]
            n466 = property on="Z-Stack" class="Bool (严格)"("DisabledEnum"=T4."Enabled" ("禁用")) -> ()  [unwired: 2 in, 2 out]
          }
        }
        n467 = disable-structure shown="启用" {
          disable-tunnel: [w980 _] -> w963
          frame Disabled {
            n468 = local read "Microscope"() -> (w983:enum16{"Miniature", "Benchtop"})
            n469 = Equal?(x=w983, y=enum16{"Miniature", "Benchtop"}."Benchtop") -> (x = y?=w981:bool)
            n470 = case shown="真" w981 {
              tunnel: [FALSE ("Enable") TRUE ("Enable")] -> w980
              frame False {
              }
              frame True {
              }
            }
          }
          frame Enabled {
          }
        }
        n471 = case shown="真" w966 {
          tunnel: w979 -> [w997 w1036]
          tunnel: w978 -> [w996 w1035]
          tunnel: [w995 w1028] -> w977
          tunnel: [w994 w1027] -> w972
          tunnel: w975 -> [w993 w1034]
          tunnel: w974 -> [w992 w1033]
          tunnel: [w987 w1032] -> w973
          tunnel: w963 -> [w986 w1022]
          frame False {
            n472 = flat-sequence {
              tunnel: [w1006] -> w991
              tunnel: [w1005] -> w990
              tunnel: [w1000] -> w989
              tunnel: [w999] -> w988
              tunnel: w997 -> [w1002]
              tunnel: w996 -> [w1001]
              tunnel: w993 -> [w1006]
              tunnel: w992 -> [w1005]
              tunnel: [w1021] -> w995
              tunnel: [w1020] -> w994
              tunnel: [w1017] -> w987
              tunnel: w991 -> [w1019]
              tunnel: w990 -> [w1018]
              tunnel: w989 -> [w1016]
              tunnel: w988 -> [w1015]
              tunnel: w986 -> [_]
              frame #0 {
                n473 = local write "Focus Flag"(FALSE ("Focus Flag")) -> ()
                n474 = xnode "读取/写入控件"("FPGA VI引用输入"=w1002, "错误输入"=w1001, "FOCUS"=FALSE ("Stop Write")) -> ("FPGA VI引用输出"=w1000:refnum<k20>, "错误输出"=w999:errorcluster)
                n475 = Wait (ms)(milliseconds to wait=u32 100 ("等待时间（毫秒）")) -> ()  [unwired: 1 out]
              }
              frame #1 {
                n476 = xnode "读取/写入控件"("FPGA VI引用输入"=w1019, "错误输入"=w1018, "Shutter"=FALSE, "Start Control"=FALSE ("Enable")) -> ("错误输出"=w1017:errorcluster)  [unwired: 1 out]
                n477 = xnode "Invoke Method"("FPGA VI引用输入"=w1016, "错误输入"=w1015, "元素数量"=u32 0, "超时(ms)"=0) -> ("FPGA VI引用输出"=w1013:refnum<k20>, "错误输出"=w1012:errorcluster, "剩余元素"=w1011:u32)  [unwired: 1 out]
                "Test Point 3" <- w1011
                n478 = xnode "Invoke Method"("FPGA VI引用输入"=w1013, "错误输入"=w1012, "元素数量"=w1011, "超时(ms)"=0) -> ("FPGA VI引用输出"=w1021:refnum<k20>, "错误输出"=w1020:errorcluster)  [unwired: 2 out]
              }
            }
          }
          frame True {
            n479 = flat-sequence {
              tunnel: w1033 -> [w1040]
              tunnel: w1034 -> [w1043]
              tunnel: w1035 -> [w1044]
              tunnel: w1036 -> [w1045]
              tunnel: [w1045] -> w1026
              tunnel: [w1044] -> w1025
              tunnel: [w1042] -> w1024
              tunnel: [w1041] -> w1023
              tunnel: w1022 -> [_]
              tunnel: [w1046] -> w1031
              tunnel: [w1049] -> w1030
              tunnel: [w1048] -> w1029
              tunnel: w1026 -> [w1049]
              tunnel: w1025 -> [w1048]
              tunnel: w1024 -> [_]
              tunnel: w1023 -> [w1046]
              tunnel: w1031 -> [w1063]
              tunnel: w1030 -> [w1058]
              tunnel: w1029 -> [w1057]
              tunnel: [w1063] -> w1032
              tunnel: [w1055] -> w1028
              tunnel: [w1054] -> w1027
              frame #0 {
                n480 = xnode "读取/写入控件"("FPGA VI引用输入"=w1043, "错误输入"=w1040, "Start Control"=TRUE ("Start"), "Shutter"=TRUE) -> ("FPGA VI引用输出"=w1042:refnum<k20>, "错误输出"=w1041:errorcluster)
                n481 = Wait (ms)(milliseconds to wait=u32 100 ("等待时间（毫秒）")) -> ()  [unwired: 1 out]
              }
              frame #1 {
                n482 = local write "Focus Flag"(TRUE ("Focus Flag")) -> ()
              }
              frame #2 {
                n483 = xnode "Invoke Method"("FPGA VI引用输入"=w1058, "错误输入"=w1057, "元素数量"=u32 0, "超时(ms)"=0) -> ("FPGA VI引用输出"=w1061:refnum<k20>, "错误输出"=w1060:errorcluster, "剩余元素"=w1059:u32)  [unwired: 1 out]
                "Test Point2" <- w1059
                n484 = xnode "Invoke Method"("FPGA VI引用输入"=w1061, "错误输入"=w1060, "元素数量"=w1059, "超时(ms)"=0) -> ("FPGA VI引用输出"=w1053:refnum<k20>, "错误输出"=w1052:errorcluster)  [unwired: 2 out]
                n485 = xnode "读取/写入控件"("FPGA VI引用输入"=w1053, "错误输入"=w1052, "FOCUS"=TRUE ("Stop Write")) -> ("FPGA VI引用输出"=w1055:refnum<k20>, "错误输出"=w1054:errorcluster)
              }
            }
          }
        }
        n486 = Merge Errors(w973, w972) -> (w971:errorcluster)
      }
      event "Z-Stack": Value Change {
        n487 = event-data() -> ()  [unwired: 1 in, 6 out]
        n488 = disable-structure shown="禁用" {
          disable-tunnel: [w1085 _] -> w1071
          frame Disabled {
            n489 = local read "Microscope"() -> (w1086:enum16{"Miniature", "Benchtop"})
            n490 = Equal?(x=w1086, y=enum16{"Miniature", "Benchtop"}."Benchtop") -> (x = y?=w1088:bool)
            n491 = case shown="假" w1088 {
              tunnel: [FALSE ("Enable") TRUE ("Enable")] -> w1085
              frame False {
              }
              frame True {
              }
            }
          }
          frame Enabled {
          }
        }
        n492 = case shown="真" "Z-Stack" {
          tunnel: w1084 -> [w1109 w1180]
          tunnel: w1083 -> [w1108 w1179]
          tunnel: [w1107 w1172] -> w1082
          tunnel: [w1106 w1171] -> w1077
          tunnel: w1080 -> [w1105 w1178]
          tunnel: w1079 -> [w1104 w1177]
          tunnel: [w1099 w1176] -> w1078
          tunnel: w1074 -> [w1095 w1163]
          tunnel: [w1092 w1166] -> w1073
          tunnel: w1071 -> [_ w1162]
          frame False {
            n493 = flat-sequence {
              tunnel: [w1119] -> w1103
              tunnel: [w1118] -> w1102
              tunnel: [w1113] -> w1101
              tunnel: [w1112] -> w1100
              tunnel: w1109 -> [w1115]
              tunnel: w1108 -> [w1114]
              tunnel: w1105 -> [w1119]
              tunnel: w1104 -> [w1118]
              tunnel: w1095 -> [w1110]
              tunnel: [w1110] -> w1094
              tunnel: w1103 -> [w1133]
              tunnel: w1102 -> [w1132]
              tunnel: w1101 -> [w1130]
              tunnel: w1100 -> [w1129]
              tunnel: [w1135] -> w1098
              tunnel: [w1134] -> w1097
              tunnel: [w1131] -> w1096
              tunnel: w1094 -> [w1121]
              tunnel: [w1121] -> w1093
              tunnel: [w1120] -> w1091
              tunnel: [w1137] -> w1099
              tunnel: [w1141] -> w1106
              tunnel: [w1143] -> w1107
              tunnel: w1098 -> [w1142]
              tunnel: w1097 -> [w1140]
              tunnel: w1096 -> [w1138]
              tunnel: w1093 -> [w1147]
              tunnel: [w1145] -> w1092
              tunnel: w1091 -> [w1139]
              frame #0 {
                n494 = local write "Focus Flag"(FALSE ("Focus Flag")) -> ()
                n495 = xnode "读取/写入控件"("FPGA VI引用输入"=w1115, "错误输入"=w1114, "FOCUS"=FALSE ("Stop Write")) -> ("FPGA VI引用输出"=w1113:refnum<k20>, "错误输出"=w1112:errorcluster)
                n496 = Wait (ms)(milliseconds to wait=u32 50 ("等待时间（毫秒）")) -> ()  [unwired: 1 out]
              }
              frame #1 {
                n497 = xnode "Invoke Method"("FPGA VI引用输入"=w1130, "错误输入"=w1129, "元素数量"=u32 0, "超时(ms)"=0) -> ("FPGA VI引用输出"=w1127:refnum<k20>, "错误输出"=w1126:errorcluster, "剩余元素"=w1125:u32)  [unwired: 1 out]
                n498 = xnode "读取/写入控件"("FPGA VI引用输入"=w1133, "错误输入"=w1132, "Start Control"=FALSE ("Enable")) -> ("FPGA VI引用输出"=w1120:refnum<k20>, "错误输出"=w1131:errorcluster)
                n499 = xnode "Invoke Method"("FPGA VI引用输入"=w1127, "错误输入"=w1126, "元素数量"=w1125, "超时(ms)"=0) -> ("FPGA VI引用输出"=w1135:refnum<k20>, "错误输出"=w1134:errorcluster)  [unwired: 2 out]
              }
              frame #2 {
                n500 = local read "Slices"() -> (w1136:u16)
                n501 = Increment(x=w1147) -> (x+1=w1144:u16)
                n502 = Greater Or Equal?(x=w1144, y=w1136) -> (x >= y?=w1146:bool)
                n503 = case shown="假" w1146 {
                  tunnel: [w1151 u16 0] -> w1145
                  tunnel: w1144 -> [w1151 _]
                  tunnel: [w1150 w1157] -> w1143
                  tunnel: w1142 -> [w1150 w1157]
                  tunnel: [w1149 w1158] -> w1141
                  tunnel: w1140 -> [w1149 w1158]
                  tunnel: w1139 -> [_ w1155]
                  tunnel: w1138 -> [w1148 w1154]
                  tunnel: [w1148 w1153] -> w1137
                  frame False {
                    n504 = property on="Move" class="Bool (严格)"("Val(Sgnl)"=TRUE ("值(信号)")) -> ()  [unwired: 2 in, 2 out]
                  }
                  frame True {
                    n505 = xnode "读取/写入控件"("FPGA VI引用输入"=w1155, "错误输入"=w1154, "Shutter"=FALSE ("Enable")) -> ("错误输出"=w1153:errorcluster)  [unwired: 1 out]
                    n506 = property on="Save" class="Bool (严格)"("DisabledEnum"=T4."Enabled" ("禁用")) -> ()  [unwired: 2 in, 2 out]
                    n507 = property on="LIVE" class="Bool (严格)"("DisabledEnum"=T4."Enabled" ("禁用")) -> ()  [unwired: 2 in, 2 out]
                  }
                }
              }
            }
          }
          frame True {
            n508 = flat-sequence {
              tunnel: w1177 -> [w1184]
              tunnel: w1178 -> [w1187]
              tunnel: w1179 -> [w1188]
              tunnel: w1180 -> [w1189]
              tunnel: [w1189] -> w1170
              tunnel: [w1188] -> w1169
              tunnel: [w1186] -> w1168
              tunnel: [w1185] -> w1167
              tunnel: [w1183] -> w1164
              tunnel: w1163 -> [w1183]
              tunnel: w1162 -> [_]
              tunnel: [w1191] -> w1175
              tunnel: [w1194] -> w1174
              tunnel: [w1193] -> w1173
              tunnel: w1170 -> [w1194]
              tunnel: w1169 -> [w1193]
              tunnel: w1168 -> [_]
              tunnel: w1167 -> [w1191]
              tunnel: [w1190] -> w1165
              tunnel: w1164 -> [w1190]
              tunnel: w1175 -> [w1209]
              tunnel: w1174 -> [w1204]
              tunnel: w1173 -> [w1203]
              tunnel: [w1209] -> w1176
              tunnel: [w1201] -> w1172
              tunnel: [w1200] -> w1171
              tunnel: [w1195] -> w1166
              tunnel: w1165 -> [w1195]
              frame #0 {
                w1181 = TRUE ("Start")
                n509 = xnode "读取/写入控件"("FPGA VI引用输入"=w1187, "错误输入"=w1184, "Start Control"=w1181, "Shutter"=w1181) -> ("FPGA VI引用输出"=w1186:refnum<k20>, "错误输出"=w1185:errorcluster)
                n510 = Wait (ms)(milliseconds to wait="Interval Time") -> ()  [unwired: 1 out]
              }
              frame #1 {
                n511 = local write "Focus Flag"(TRUE ("Focus Flag")) -> ()
              }
              frame #2 {
                n512 = xnode "Invoke Method"("FPGA VI引用输入"=w1204, "错误输入"=w1203, "元素数量"=u32 0, "超时(ms)"=0) -> ("FPGA VI引用输出"=w1207:refnum<k20>, "错误输出"=w1206:errorcluster, "剩余元素"=w1205:u32)  [unwired: 1 out]
                n513 = xnode "Invoke Method"("FPGA VI引用输入"=w1207, "错误输入"=w1206, "元素数量"=w1205, "超时(ms)"=0) -> ("FPGA VI引用输出"=w1199:refnum<k20>, "错误输出"=w1198:errorcluster)  [unwired: 2 out]
                n514 = xnode "读取/写入控件"("FPGA VI引用输入"=w1199, "错误输入"=w1198, "FOCUS"=TRUE ("Stop Write")) -> ("FPGA VI引用输出"=w1201:refnum<k20>, "错误输出"=w1200:errorcluster)
              }
            }
          }
        }
        n515 = case shown="真" "Z-Stack" {
          frame False {
          }
          frame True {
          }
        }
        n516 = Merge Errors(w1078, w1077) -> (w1076:errorcluster)
      }
      event "Pixel/Line", "Line": Value Change {
        n517 = event-data() -> ()  [unwired: 1 in, 6 out]
        n518 = xnode "读取/写入控件"("FPGA VI引用输入"=w1224, "错误输入"=w1223, "FOCUS"=FALSE) -> ("FPGA VI引用输出"=w1217:refnum<k20>, "错误输出"=w1214:errorcluster)
        n519 = flat-sequence {
          tunnel: w1217 -> [w1239]
          tunnel: [w1239] -> w1216
          tunnel: [w1238] -> w1215
          tunnel: w1214 -> [w1238]
          frame #0 {
            n520 = Wait (ms)(milliseconds to wait=u32 5 ("等待时间（毫秒）")) -> ()  [unwired: 1 out]
          }
        }
        n521 = xnode "Invoke Method"("FPGA VI引用输入"=w1216, "错误输入"=w1215, "元素数量"=u32 0, "超时(ms)"=0) -> ("FPGA VI引用输出"=w1227:refnum<k20>, "错误输出"=w1228:errorcluster, "剩余元素"=w1225:u32)  [unwired: 1 out]
        n522 = xnode "Invoke Method"("FPGA VI引用输入"=w1227, "错误输入"=w1228, "元素数量"=w1225, "超时(ms)"=0) -> ("FPGA VI引用输出"=w1213:refnum<k20>, "错误输出"=w1212:errorcluster)  [unwired: 2 out]
        n523 = local read "LIVE"() -> (w1210:bool)
        n524 = case shown="假" w1210 {
          tunnel: [w1232 w1236] -> w1221
          tunnel: [w1231 w1235] -> w1220
          tunnel: w1213 -> [w1232 w1234]
          tunnel: w1212 -> [w1231 w1233]
          frame False {
          }
          frame True {
            n525 = xnode "读取/写入控件"("FPGA VI引用输入"=w1234, "错误输入"=w1233, "FOCUS"=TRUE) -> ("FPGA VI引用输出"=w1236:refnum<k20>, "错误输出"=w1235:errorcluster)
          }
        }
      }
      event "Stop": Value Change {
        n526 = event-data() -> ()  [unwired: 1 in, 3 out]
        n527 = xnode "Invoke Method"("FPGA VI引用输入"=w1251, "错误输入"=w1250) -> ("FPGA VI引用输出"=w1245:refnum<k20>, "错误输出"=w1244:errorcluster)
        n528 = xnode "Invoke Method"("FPGA VI引用输入"=w1245, "错误输入"=w1244) -> ("FPGA VI引用输出"=w1243:refnum<k20>, "错误输出"=w1242:errorcluster)
        n529 = xnode "Invoke Method"("FPGA VI引用输入"=w1243, "错误输入"=w1242) -> ("FPGA VI引用输出"=w1253:refnum<k20>, "错误输出"=w1252:errorcluster)
        "Power Stop" <- TRUE ("Power Stop")
      }
    }
  }
  n530 = local read "Rolling Average"() -> (w33:dbl)
  n531 = Obtain Queue(max queue size (-1, unlimited)=w33, name (unnamed)="Rolling Init" ("名称（未命名）"), element data type=dbl[][] [] ("x/y")) -> (queue out=w45:refnum<queue>, error out=w46:errorcluster)  [unwired: 2 in, 1 out]
  n532 = call "IMAQ Create"("Image Name"="ROI Mask", "Image Type"=w3) -> ("New Image"=w2:T1, "error out"=w1:errorcluster)  [unwired: 3 in]
  n533 = call "IMAQ Create"("Image Name"="Rolling", "Image Type"=w35) -> ("New Image"=w39:T1)  [unwired: 3 in, 1 out]
  n534 = call "IMAQ Create"("Image Name"="Display-IMAQ", "Image Type"=w9) -> ("New Image"=w8:T1)  [unwired: 3 in, 1 out]
  n535 = call "IMAQ Create"("Image Name"="92", "Image Type"=w15) -> ("New Image"=w13:T1, "error out"=w12:errorcluster)  [unwired: 3 in]
  n536 = Initialize Array(0.0 ("元素"), w38, w38) -> (w36:dbl[][])
  n537 = while {
    shift-right: [w1271] -> _
    shift-left: w36 -> [w1272]
    tunnel: w39 -> [w1270]
    shift-right: [w1269] -> w40
    shift-left: w45 -> [w1267]
    shift-right: [w1268] -> w41
    shift-left: w46 -> [w1266]
    shift-right: [w1265] -> _
    shift-left: 1.0 ("Rolling Average") -> [w1264]
    tunnel: w21 -> [w1262]
    shift-right: [w1259] -> _
    shift-left: u16 0 -> [w1260]
    tunnel: w13 -> [w1258]
    tunnel: w12 -> [w1257]
    tunnel: w8 -> [w1256]
    tunnel: w2 -> [w1255]
    tunnel: w1 -> [w1254]
    i -> [w1263]
    stop <- w1275 stop-if-true
    n538 = Dequeue Element(queue=w1262) -> (queue out=w1261:refnum<queue>, element=w1273:u16[][], error out=w1274:errorcluster)  [unwired: 2 in, 1 out]
    n539 = case shown="无错误" w1274 {
      tunnel: [_ TRUE] -> w1275
      tunnel: w1273 -> [w1290 _]
      tunnel: w1272 -> [w1297 _]
      tunnel: [w1280 dbl[][] [] ("x/y")] -> w1271
      tunnel: w1270 -> [w1292 _]
      tunnel: [w1302 w1385] -> w1269
      tunnel: [w1295 w1384] -> w1268
      tunnel: w1267 -> [w1300 w1385]
      tunnel: w1266 -> [w1299 w1384]
      tunnel: [w1298 w1383] -> w1265
      tunnel: w1264 -> [w1301 w1383]
      tunnel: w1263 -> [w1296 _]
      tunnel: w1261 -> [w1294 _]
      tunnel: w1260 -> [w1288 _]
      tunnel: [w1287 u16 0] -> w1259
      tunnel: w1258 -> [w1285 _]
      tunnel: w1257 -> [w1284 _]
      tunnel: w1256 -> [w1281 _]
      tunnel: w1255 -> [w1278 _]
      tunnel: w1254 -> [w1276 _]
      frame No Error {
        n540 = local read "Pulse Number"() -> (w1283:enum16{"SP", "DP"})
        n541 = Get Queue Status(queue=w1294) -> (# elements in queue=→"Memory":i32)  [unwired: 2 in, 7 out]
        n542 = Increment(x=w1288) -> (x+1=w1287:u16)
        "Total Frames" <- w1287
        n543 = call "sub_数组奇数行转置.vi"("Pulse Number"=w1283, "Input"=w1290) -> ("output"=w1289:u16[][])
        n544 = Subtract(x=u16 65535, y=w1289) -> (x-y=w1282:u16[][])
        n545 = case shown="假" "Rolling" {
          tunnel: [w1342 w1363] -> w1280
          tunnel: [w1341 w1362] -> w1302
          tunnel: w1301 -> [w1340 _]
          tunnel: w1300 -> [w1341 w1361]
          tunnel: w1299 -> [w1344 w1360]
          tunnel: [w1340 w1359] -> w1298
          tunnel: w1297 -> [w1342 w1358]
          tunnel: w1296 -> [_ w1357]
          tunnel: [w1343 w1356] -> w1295
          tunnel: w1282 -> [w1346 w1355]
          tunnel: w1292 -> [_ w1354]
          tunnel: [w1345 w1348] -> w1279
          tunnel: w1281 -> [w1339 _]
          frame False {
            n546 = call "IMAQ ArrayToImage"("Image Pixels (U16)"=w1346, "error in (no error)"=w1344, "Image"=w1339) -> ("error out"=w1343:errorcluster, "Image Out"=w1345:T1)  [unwired: 7 in]
          }
          frame True {
            n547 = case shown="真" "Rolling Queue Flag" {
              tunnel: [w1367 w1373] -> w1351
              tunnel: [w1365 w1372] -> w1353
              tunnel: [w1366 w1380] -> w1359
              tunnel: "Rolling Average" -> [w1366 w1380]
              tunnel: w1361 -> [w1367 w1375]
              tunnel: w1360 -> [w1365 w1374]
              tunnel: [w1364 w1377] -> w1352
              tunnel: w1358 -> [w1364 _]
              tunnel: w1357 -> [_ w1369]
              frame False {
              }
              frame True {
                w1378 = 2048 ("维数大小")
                n548 = Release Queue(queue=w1375, error in (no error)=w1374) -> ()  [unwired: 1 in, 3 out]
                n549 = local write "Rolling Queue Flag"(FALSE ("Rolling Queue Flag")) -> ()
                n550 = Number To Decimal String(number=w1369) -> (decimal integer string=w1370:string)  [unwired: 1 in]
                n551 = Obtain Queue(max queue size (-1, unlimited)=w1380, name (unnamed)=w1370, element data type=dbl[][] [] ("x/y")) -> (queue out=w1376:refnum<queue>, error out=w1371:errorcluster)  [unwired: 2 in, 1 out]
                n552 = Initialize Array(0.0 ("元素"), w1378, w1378) -> (w1377:dbl[][])
                n553 = Flush Queue(queue=w1376, error in (no error)=w1371) -> (queue out=w1373:refnum<queue>, error out=w1372:errorcluster)  [unwired: 1 out]
              }
            }
            n554 = call "sub_rolling average.vi"("Raw Data"=w1355, "错误输入（无错误）"=w1353, "队列输入"=w1351, "移位in"=w1352, "Image Create"=w1354) -> ("错误输出"=w1356:errorcluster, "队列输出"=w1362:refnum<queue>, "移位out"=w1363:dbl[][], "Image Display"=w1348:T1, "队列中元素数量"=→"Queue Number":i32)  [unwired: 2 in]
          }
        }
        "Image" <- w1279
        n555 = case shown="真" "ROI Statistic" {
          tunnel: w1279 -> [_ w1308]
          tunnel: w1278 -> [_ w1309]
          tunnel: w1276 -> [_ w1307]
          frame False {
          }
          frame True {
            n556 = property on="Image" class="ImageControl"() -> ("ROI"=w1310:T5)  [unwired: 2 in, 2 out]
            n557 = call "ROI统计量16bit.vi"("error in (no error)"=w1307, "ROI Descriptor"=w1310, "Image Mask"=w1309, "Image"=w1308) -> ("统计量"=w1311:sgl[])  [unwired: 5 in, 2 out]
            n558 = Index Array(array=w1311, index #1=0 ("索引"), index #2=1 ("索引"), index #3=2 ("索引"), index #4=3 ("索引")) -> (element #1=w1305:sgl, element #2=→"Variation":sgl, element #3=→"Minimal":sgl, element #4=→"Maximal":sgl)
            n559 = Subtract(x=w1305, y=sgl 32751.0) -> (x-y=→"Mean Value" →"波形图表":sgl)
          }
        }
        n560 = disable-structure shown="启用" {
          disable-tunnel: "Calculate Phase shift" -> [w1322 _]
          disable-tunnel: w1279 -> [w1321 _]
          disable-tunnel: w1285 -> [w1320 _]
          disable-tunnel: w1284 -> [w1319 _]
          frame Enabled {
            n561 = case shown="真" w1322 {
              tunnel: w1321 -> [_ w1325]
              tunnel: w1320 -> [_ w1324]
              tunnel: w1319 -> [_ w1323]
              frame False {
              }
              frame True {
                n562 = property on="Image" class="ImageControl"() -> ("ROI"=w1328:T5)  [unwired: 2 in, 2 out]
                n563 = Unbundle By Name(w1328) -> ("Global Rectangle"=w1330:i32[])
                n564 = call "sub_转换成偶数数组.vi"("输入数组"=w1330) -> ("输出数组"=w1329:i32[])
                n565 = call "IMAQ Extract 2"("Optional Rectangle"=w1329, "error in (no error)"=w1323, "Image Dst"=w1324, "Image Src"=w1325) -> ("error out"=w1333:errorcluster, "Image Dst Out"=w1332:T1)  [unwired: 6 in]
                n566 = call "IMAQ ImageToArray"("error in (no error)"=w1333, "Image"=w1332) -> ("Image Pixels (U16)"=w1331:u16[][])  [unwired: 2 in, 4 out]
                n567 = To Double Precision Float(number=w1331) -> (double precision float=w1334:dbl[][])
                n568 = Subtract(x=w1334, y=32768.0) -> (x-y=w1336:dbl[][])
                n569 = call "sub_提取奇偶行2.vi"("数组"=w1336) -> ("奇数行一维数组"=w1338:dbl[], "偶数行一维数组"=w1337:dbl[])  [unwired: 5 in]
                n570 = call "sub_互相关.vi"("互相关点数"="互相关点数", "y"=w1337, "x"=w1338) -> ("中心偏移"=→"中心偏移":i32)  [unwired: 2 in, 2 out]
              }
            }
          }
          frame Disabled {
          }
        }
      }
      frame Error {
      }
    }
  }
  n571 = xnode "关闭FPGA VI引用"("FPGA VI引用输入"=w57, "错误输入"=w56) -> ()  [unwired: 1 out]
  n572 = Release Queue(queue=w32, error in (no error)=w73) -> ()  [unwired: 1 in, 3 out]
  n573 = Release Queue(queue=w21, error in (no error)=w20) -> ()  [unwired: 1 in, 3 out]
  n574 = Release Queue(queue=w40, error in (no error)=w41) -> ()  [unwired: 1 in, 3 out]
  n575 = xnode "关闭FPGA VI引用"("FPGA VI引用输入"=w72, "错误输入"=w71) -> ()  [unwired: 1 out]
